vi "Periodic Tasks.vi"(8 "error in":errorcluster) -> ()   [LabVIEW 2018]
doc: "This VI runs in parallel to other tasks. It can contain as many user-defined periodic loops as you need. These can carry out PID or other sorts of timed response."
uses:
  <vilib>/Rock Robotics/WPI/ThirdParty/Phoenix-LabVIEW/Motor Controller/Controls/CTRE_Phoenix_MotorControl_ControlMode.ctl
  <vilib>/Rock Robotics/WPI/Utilities/WPI_GetSetVariantRefNum.vi
  <vilib>/Rock Robotics/Network Tables/NT Write Boolean Array.vi
  <vilib>/Rock Robotics/Network Tables/NT Write Numeric Array.vi
  <vilib>/Rock Robotics/WPI/Dashboard/Steer Command Global.vi
  <vilib>/Rock Robotics/WPI/Dashboard/Drive Command Global.vi
  Robot Global Data.vi
  <vilib>/Rock Robotics/Network Tables/NT Write Boolean.vi
  <vilib>/Rock Robotics/WPI/RobotDrive/WPI_RobotDriveMecanumDrive_Cartesian.vi
  <vilib>/Rock Robotics/WPI/ThirdParty/Phoenix-LabVIEW/Motor Controller/Get/CTRE_Phoenix_MotorController_GetAnalogData.vi
  <vilib>/Rock Robotics/Network Tables/NT Write Number.vi
  <vilib>/Rock Robotics/Network Tables/NT Read Number.vi
  <vilib>/Rock Robotics/WPI/Dashboard/Valid Target Global.vi
panel:
  out "TargetValid":bool
  out "DriveCommand":dbl(knob)=-0.0 scale=0.0..1.0
  in  "MaxDrive":dbl(slide)=0.20072992700729927 min=0.0 max=1.0 step=0.01 scale=0.0..1.0
  in  "DriveK":dbl(slide)=0.26277372262773724 min=0.0 max=1.0 step=0.05 scale=0.0..1.0
  in  "Limelight Goal Area":dbl(slide)=14.872262773722628 min=0.1 max=25.0 step=0.25 scale=0.0..25.0
  out "SteerCommand":dbl(knob) scale=-1.0..1.0
  in  "AimDeadband":dbl min=0.0 max=10.0 step=0.25
  in  "MinSteerCommand":dbl(slide)=0.02717391304347826 min=0.0 max=0.5 step=0.05 scale=0.0..0.5
  in  "SteeringK":dbl(slide)=0.007246376811594203 min=0.0 max=0.25 step=0.01 scale=0.0..0.25
  in  "Jack speed 3-2":dbl=-1.0
  in  "Jack drive 1-2":dbl=-0.75
  in  "Jack speed 2-2":dbl=1.0
  in  "Jack speed 1-2":dbl=1.0
  in  "Arm speed-2":dbl=-0.41
  in  "Pre Climb 2":i32=146
  in  "Load Cargo":i32=385
  in  "Arm speed":dbl=-0.55
  in  "Jack speed 1":dbl=1.0
  in  "Jack speed 2":dbl=1.0
  in  "Jack drive 1":dbl=-0.75
  in  "Jack speed 3":dbl=-1.0
  in  "Pre Climb":i32=80
  in  "Release Time":i32=7
  in  "Grab Drive Time":i32=7
  in  "Grab Wait Time":i32=2
  in  "Grab Time":i32=5
  in  "Home":i32=70
  in  "C High":i32=890
  in  "C Med":i32=540
  in  "C Low":i32=230
  in  "H High":i32=809
  in  "H Med":i32=475
  in  "H Low":i32=140
  out "Jack PO":dbl
  out "Arm PO":dbl
  out "Arm position":i32=55
  # "Climb 2 Case Values"
  # "Arm Actuators"
  # "Jack Mech."
  # "Jack Wheels"
  # "In pre climb cases add about 5% drive forward"
  # "Climb Case Values"
  # "Arm Actuators"
  # "Jack Mech."
  # "Jack Wheels"
  # "Grab and Release Times and Values\n                 In State Machine"
  # "State Machine Values for Positions"
  # "Proto Values Before Heartland"
  # "Pre Climb 2 146"
  # "H Low 171\nH Med 475\nH High 809"
  # "C Low 230\nC Med 540\nC High 890"
  # "Load Cargo 385\nHome 70\nPre Climb 80"
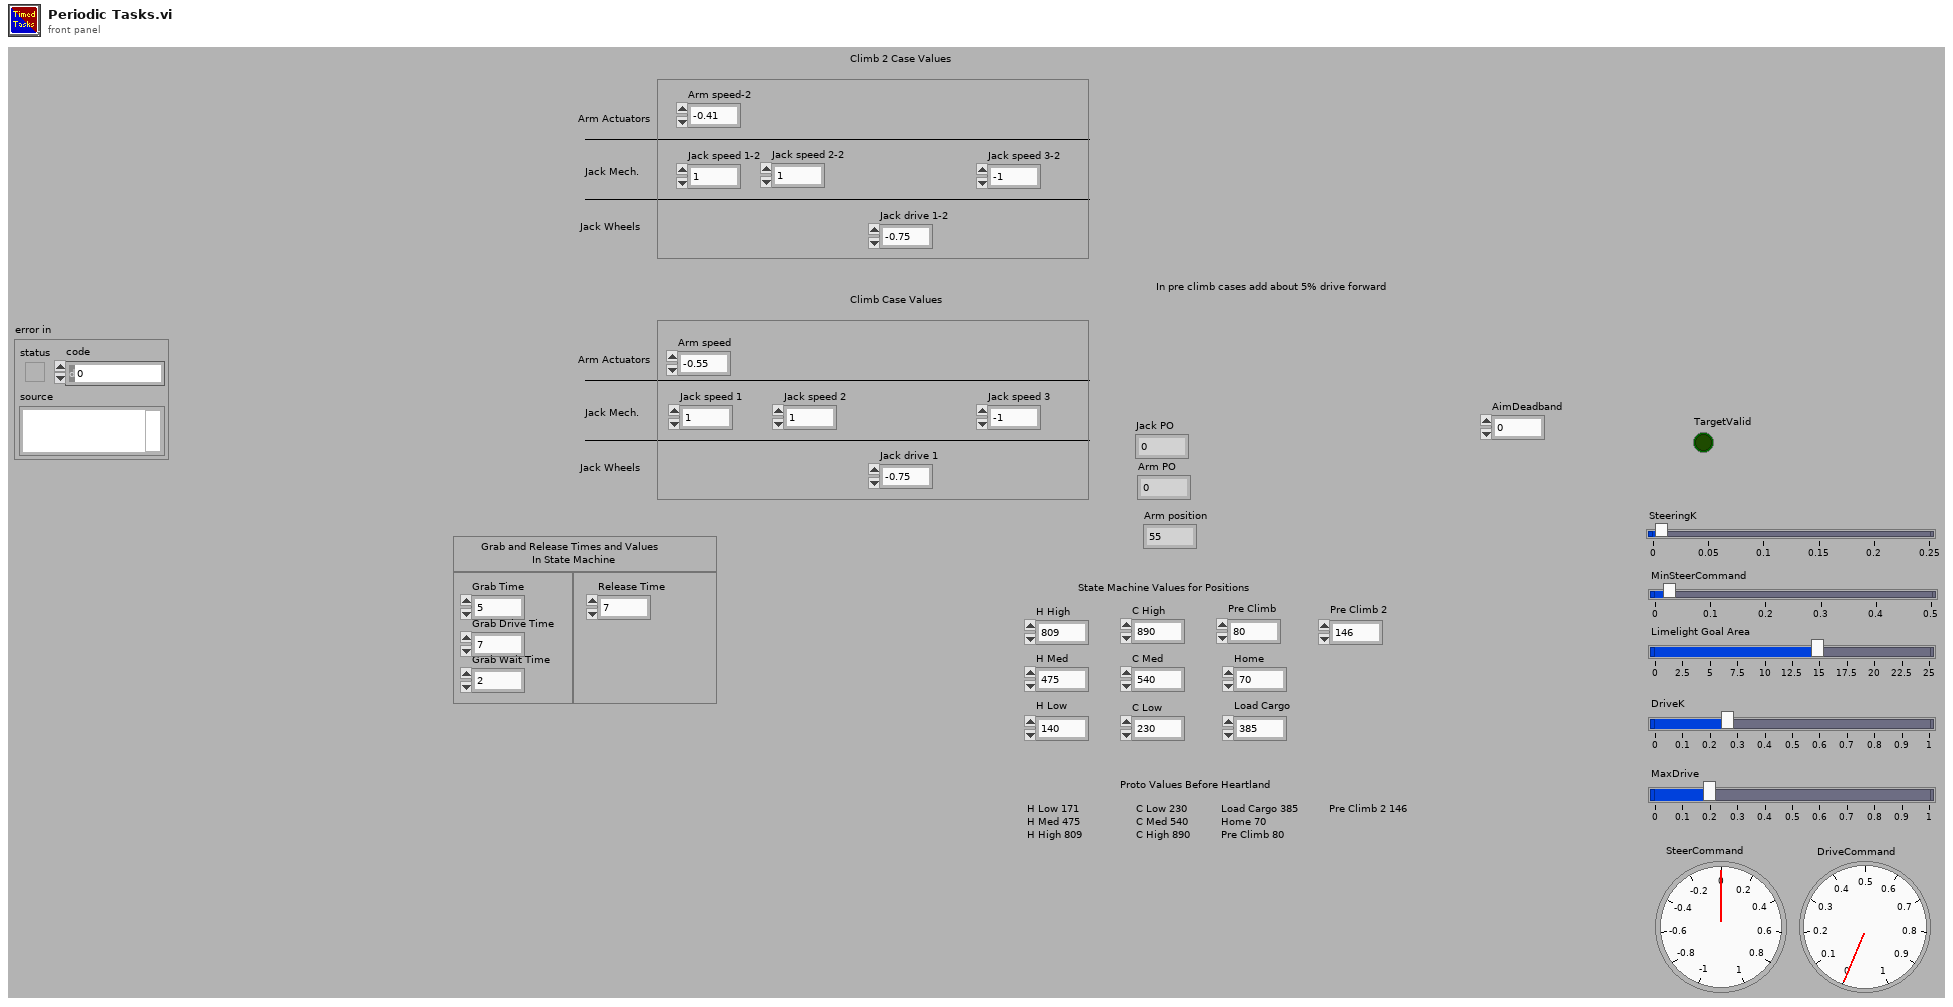
[diagram p1: front panel]
types:
  T1 = enum16{"Wait", "H.Low", "H.Med", "H.High", "C.Low", "C.Med", "C.High", "Home", "Pull Out Grab", "Pull Out Release", "Pre Climb", "Upward Travel", "Extra Jack Time", "Forward Travel", "Jack Retrieval", "Load Cargo", "Pre Climb 2", "Upward Travel 2", "Extra Jack Time 2", "Forward Travel 2", "Jack Retrieval 2"}
  T2 = typedef "WPI_DriverStationRobotMode2.ctl" = enum16{"Autonomous Disabled", "Autonomous Enabled", "Teleop Disabled", "Teleop Enabled", "Disconnected", "Finish", "Test Disabled", "Test Enabled", "Emergency Stopped"}
  T3 = typedef "WPI_MotorControlDeviceRef.ctl" = cluster{"DeviceStatus":errorcluster, "Type":T4, "PWM":cluster{"PWM Channel":T5, "DeadBand":T6}, "CAN":cluster{"Device Number":u8, "SetOutput VI Ref":variant, "GetOutput VI Ref":variant, "Enable VI Ref":variant, "Disable VI Ref":variant, "Data":variant}, "Invert":bool, "DIO PWM":cluster{"PWM \"Enable\" Channel":T5, "DIOChannel":T7, "PWM Rate":dbl}}
  T4 = typedef "WPI_MotorControlType.ctl" = enum16{"PWM", "CAN", "DIO PWM"}
  T5 = typedef "FPGA_DIOPWMChannel.ctl" = enum8{"PWM 0", "PWM 1", "PWM 2", "PWM 3", "PWM 4", "PWM 5", "PWM 6", "PWM 7", "PWM 8", "PWM 9", "PWM MXP 0", "PWM MXP 1", "PWM MXP 2", "PWM MXP 3", "PWM MXP 4", "PWM MXP 5", "PWM MXP 6", "PWM MXP 7", "PWM MXP 8", "PWM MXP 9", "Invalid"}
  T6 = typedef "WPI_PWMDeadband.ctl" = cluster{"Name":string, "maxPositivePwm":i32, "minPositivePwm":i32, "centerPwm":i32, "maxNegativePwm":i32, "minNegativePwm":i32, "angularRange":u16}
  T7 = typedef "FPGA_DIOChannel.ctl" = enum8{"DIO 0", "DIO 1", "DIO 2", "DIO 3", "DIO 4", "DIO 5", "DIO 6", "DIO 7", "DIO 8", "DIO 9", "DIO MXP 0", "DIO MXP 1", "DIO MXP 2", "DIO MXP 3", "DIO MXP 4", "DIO MXP 5", "DIO MXP 6", "DIO MXP 7", "DIO MXP 8", "DIO MXP 9", "DIO MXP 10", "DIO MXP 11", "DIO MXP 12", "DIO MXP 13", "DIO MXP 14", "DIO MXP 15", "SPI Port CS1", "SPI Port CS2", "SPI Port CS3", "SPI Port MISO", "SPI Port MOSI", "Invalid"}
  T8 = typedef "WPI_JoystickDevRef.ctl" = cluster{"Device":T9}
  T9 = typedef "WPI_JoystickDeviceEnum.ctl" = enum16{"USB 0", "USB 1", "USB 2", "USB 3", "USB 4", "USB 5"}
  T10 = typedef "CTRE_Phoenix_MotorControl_ControlMode.ctl" = u16
  T11 = typedef "WPI_RobotDriveDevRef.ctl" = cluster{"DevStatus":errorcluster, "Motors[]":T3[], "Square Inputs":bool, "Max Output":dbl}
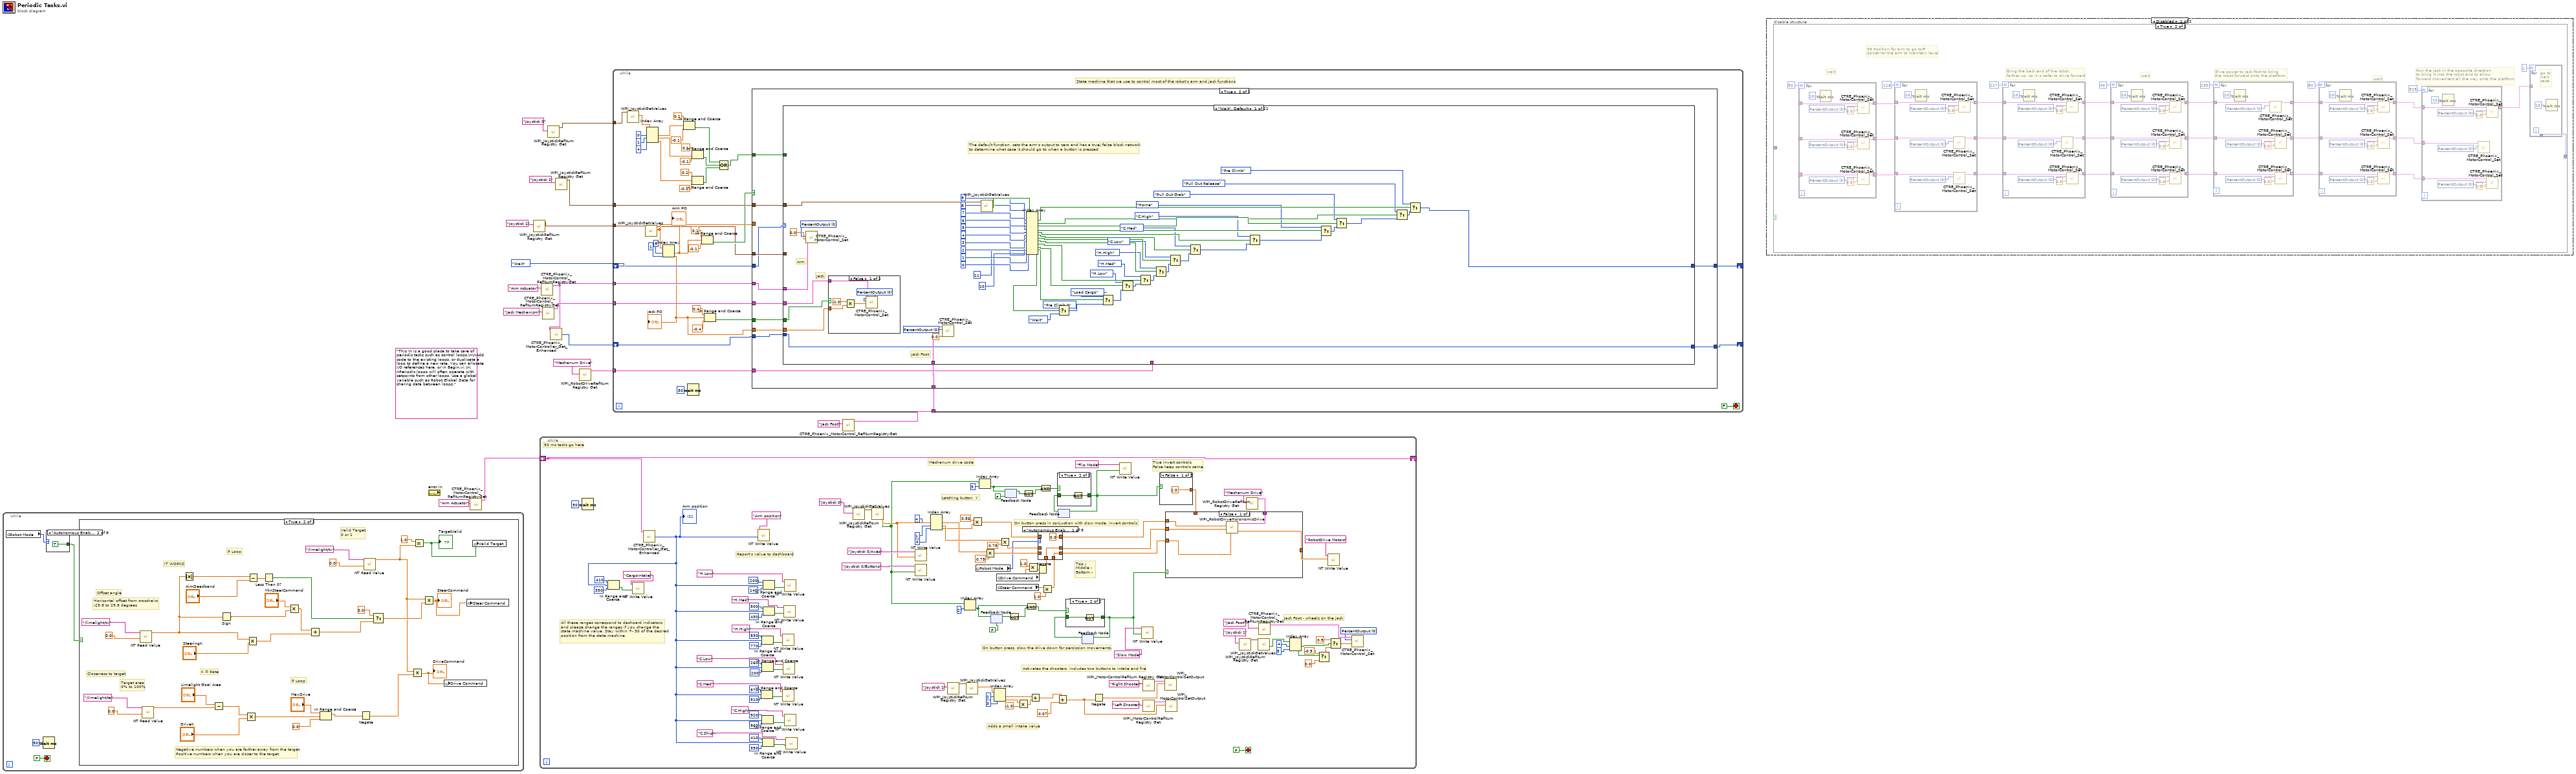
[diagram p0: block diagram]
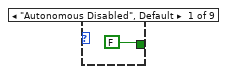
[diagram p2: hidden frame]
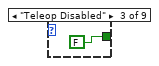
[diagram p3: hidden frame]
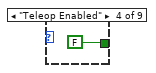
[diagram p4: hidden frame]
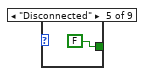
[diagram p5: hidden frame]
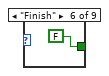
[diagram p6: hidden frame]
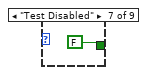
[diagram p7: hidden frame]
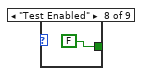
[diagram p8: hidden frame]
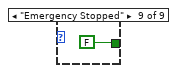
[diagram p9: hidden frame]
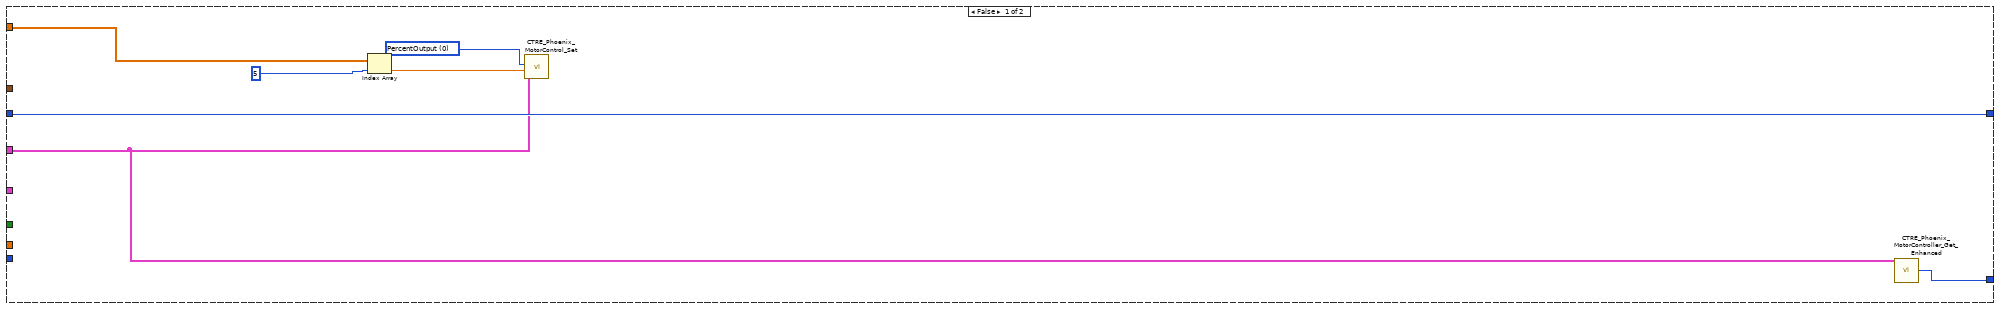
[diagram p13: hidden frame]
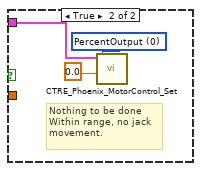
[diagram p14: hidden frame]
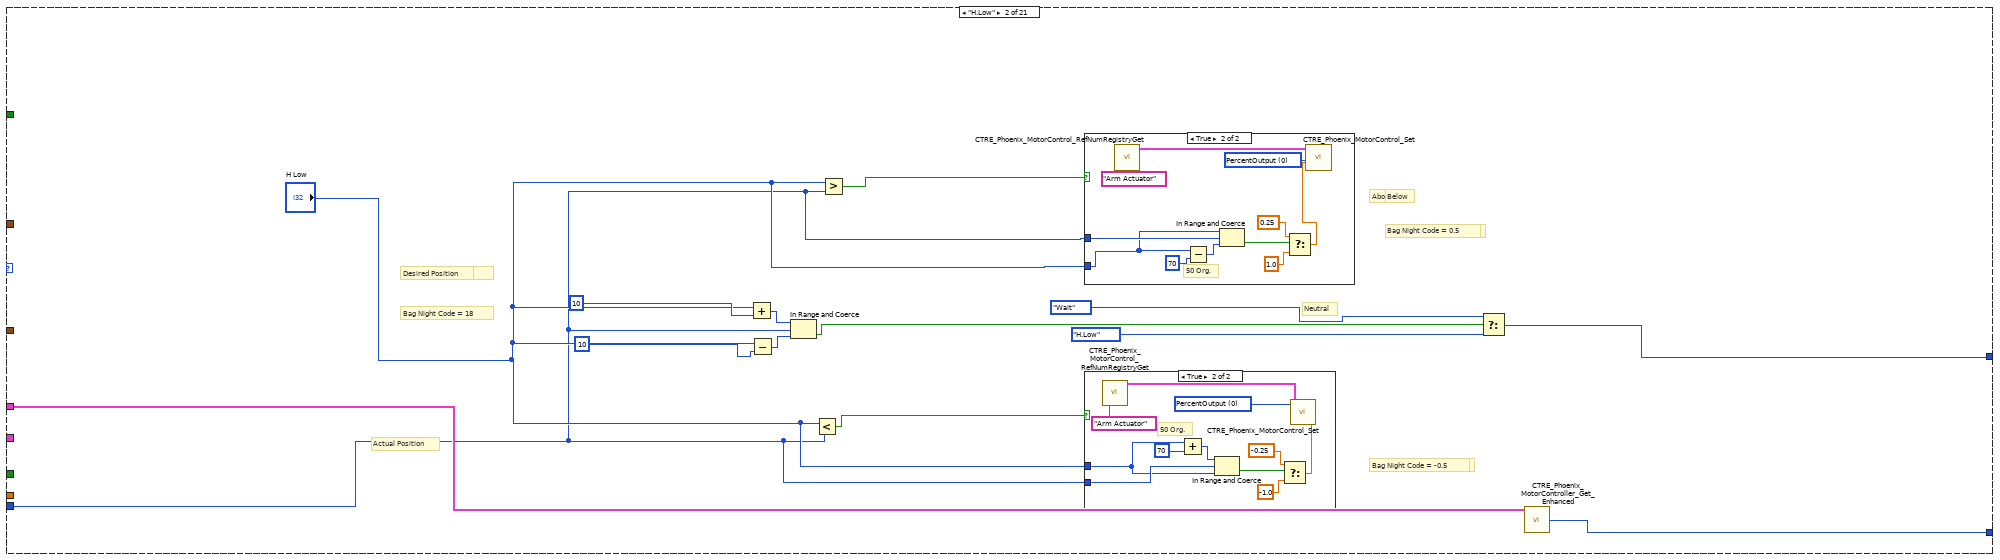
[diagram p15: hidden frame]
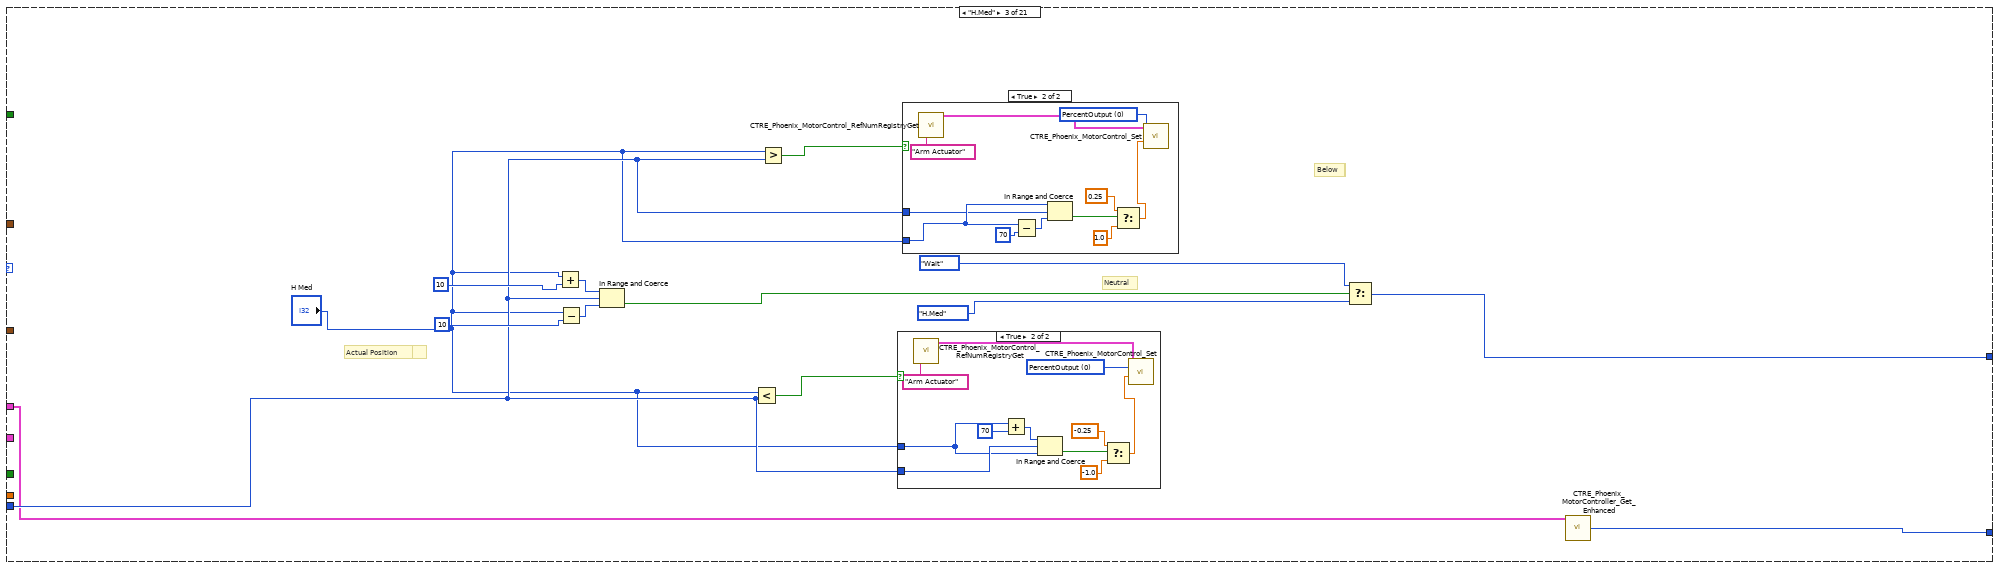
[diagram p18: hidden frame]
diagram:
  (unwired) "This VI is a good place to take care of periodic tasks such as control loops.\n\nAdd code to the existing loops, or duplicate a loop to define a new rate. You can allocate I/O references here, or in Begin.vi.\n\nPeriodic loops will often operate with setpoints from other loops. Use a global variable such as Robot Global Data for sharing data between loops."
  n1 = while {
    stop <- FALSE stop-if-true
    n2 = global read "Robot Global Data.vi" "Robot Mode"() -> (w21:T2)
    n3 = Wait (ms)(milliseconds to wait=u32 50) -> ()  [unwired: 1 out]
    n4 = case shown="\"Autonomous Enabled\"" w21 {
      tunnel: [FALSE TRUE FALSE FALSE FALSE FALSE FALSE FALSE FALSE] -> w22
      frame "Autonomous Disabled", Default {
      }
      frame "Autonomous Enabled" {
      }
      frame "Teleop Disabled" {
      }
      frame "Teleop Enabled" {
      }
      frame "Disconnected" {
      }
      frame "Finish" {
      }
      frame "Test Disabled" {
      }
      frame "Test Enabled" {
      }
      frame "Emergency Stopped" {
      }
    }
    n5 = case shown="True" w22 {
      frame False {
      }
      frame True {
        # "IT WORKS"
        # "Offset angle"
        # "Closeness to target"
        # "K = Rate"
        # "P Loop"
        # "P Loop"
        # "Negative numbers when you are farther away from the target\nPositive numbers when you are closer to the target"
        # "Valid Target\n0 or 1"
        # "Target area\n0% to 100%"
        # "Horizontal offset from crosshairs\n-29.8 to 29.8 degrees"
        n6 = call-poly <vilib>:"NT Read Value.vi"("Default Value"=0.0, "Name"="/limelight/tx") -> ("Numeric"=w38:dbl)  [unwired: 8 in, 1 out]
        n7 = call-poly <vilib>:"NT Read Value.vi"("Default Value"=0.0, "Name"="/limelight/ta") -> ("Numeric"=w46:dbl)  [unwired: 8 in, 1 out]
        n8 = Absolute Value(x=w38) -> (abs(x)=w60:dbl)
        n9 = Subtract(x="Limelight Goal Area", y=w46) -> (x-y=w44:dbl)
        n10 = Sign(1:w38) -> (0:w48:dbl)
        n11 = Multiply(x=w44, y="DriveK") -> (x*y=w43:dbl)
        n12 = Multiply(x=w38, y="SteeringK") -> (x*y=w57:dbl)
        n13 = Subtract(x=w60, y="AimDeadband") -> (x-y=w62:dbl)
        n14 = Less Than 0?(x=w62) -> (x < 0?=w63:bool)
        n15 = Multiply(x="MinSteerCommand", y=w48) -> (x*y=w59:dbl)
        n16 = Add(x=w59, y=w57) -> (x+y=w37:dbl)
        n17 = In Range and Coerce(upper limit="MaxDrive", x=w43, lower limit=0.0) -> (coerced(x)=w40:dbl)  [unwired: 1 out]
        n18 = Negate(x=w40) -> (-x=w39:dbl)
        n19 = call-poly <vilib>:"NT Read Value.vi"("Default Value"=0.0, "Name"="/limelight/tv") -> ("Numeric"=w36:dbl)  [unwired: 8 in, 1 out]
        n20 = Select(t=0.0, s=w63, f=w37) -> (s? t:f=w50:dbl)
        n21 = Multiply(x=w36, y=w39) -> (x*y=w32:dbl)
        "DriveCommand" <- w32
        n22 = Equal?(x=1.0, y=w36) -> (x = y?=w34:bool)
        "TargetValid" <- w34
        n23 = Multiply(x=w36, y=w50) -> (x*y=w33:dbl)
        "SteerCommand" <- w33
        n24 = global write "Drive Command Global.vi" "Drive Command"(w32) -> ()
        n25 = global write "Steer Command Global.vi" "Steer Command"(w33) -> ()
        n26 = global write "Valid Target Global.vi" "Valid Target"(w34) -> ()
      }
    }
  }
  n27 = call <vilib>:"CTRE_Phoenix_MotorControl_RefNumRegistryGet.vi"("refnum name"="Arm Actuator") -> ("PhoenixMotorControlDevRef"=w17:T3)  [unwired: 9 in, 1 out]
  n28 = call <vilib>:"WPI_JoystickRefNum Registry Get.vi"("refnum name"="Joystick 1") -> ("JoystickDevRef"=w13:T8)  [unwired: 9 in, 1 out]
  n29 = while {
    shift-right: [w113] -> _
    shift-left: w17 -> [w113]
    stop <- FALSE stop-if-true
    w90 = T10 0 items=["PercentOutput"=0, "Position"=1, "Velocity"=2, "Current"=3, "Follower"=5, "MotionProfile"=6, "MotionMagic"=7, "MotionProfileArc"=10, "Disabled"=15] ("Control Mode")
    # "Top -\nMiddle -\nBottom -"
    # "On button press in conjuction with slow mode, invert controls"
    # "Latching button  Y"
    # "True invert controls\nFalse keep controls same"
    # "Jack Foot - wheels on the jack"
    # "All these ranges correspond to dashoard indicators\nand please change the ranges if you change the \nstate machine value. Stay within +- 30 of the desired\nposition from the state machine."
    # "Adds a small intake value"
    # "On button press, slow the drive down for percission movements."
    # "Report's value to dashboard"
    # "Mechanum drive code"
    # "Activates the shooters, includes two buttons to intake and fire"
    # "50 ms tasks go here"
    n30 = Wait (ms)(milliseconds to wait=u32 50) -> ()  [unwired: 1 out]
    n31 = call-poly <vilib>:"CTRE_Phoenix_MotorController_Get_Enhanced.vi"("PhoenixMotorControlDevRef"=w113) -> ("AnalogInRaw"=w121:i32)  [unwired: 10 in, 4 out]
    "Arm position" <- w121
    n32 = In Range and Coerce(upper limit=410, x=w121, lower limit=350) -> (In Range?=w118:bool)  [unwired: 1 out]
    n33 = call-poly <vilib>:"NT Write Value.vi"("Boolean"=w118, "Name"="CargoIntake") -> ()  [unwired: 9 in, 1 out]
    n34 = call-poly <vilib>:"NT Write Value.vi"("Numeric"=w121, "Name"="Arm position") -> ()  [unwired: 9 in, 1 out]
    n35 = In Range and Coerce(upper limit=570, x=w121, lower limit=510) -> (In Range?=w136:bool)  [unwired: 1 out]
    n36 = In Range and Coerce(upper limit=260, x=w121, lower limit=200) -> (In Range?=w135:bool)  [unwired: 1 out]
    n37 = In Range and Coerce(upper limit=830, x=w121, lower limit=770) -> (In Range?=w134:bool)  [unwired: 1 out]
    n38 = In Range and Coerce(upper limit=920, x=w121, lower limit=860) -> (In Range?=w138:bool)  [unwired: 1 out]
    n39 = In Range and Coerce(upper limit=410, x=w121, lower limit=350) -> (In Range?=w137:bool)  [unwired: 1 out]
    n40 = In Range and Coerce(upper limit=200, x=w121, lower limit=140) -> (In Range?=w132:bool)  [unwired: 1 out]
    n41 = In Range and Coerce(upper limit=500, x=w121, lower limit=430) -> (In Range?=w133:bool)  [unwired: 1 out]
    n42 = call-poly <vilib>:"NT Write Value.vi"("Boolean"=w134, "Name"="H.High") -> ()  [unwired: 9 in, 1 out]
    n43 = call-poly <vilib>:"NT Write Value.vi"("Boolean"=w136, "Name"="C.Med") -> ()  [unwired: 9 in, 1 out]
    n44 = call-poly <vilib>:"NT Write Value.vi"("Boolean"=w135, "Name"="C.Low") -> ()  [unwired: 9 in, 1 out]
    n45 = call-poly <vilib>:"NT Write Value.vi"("Boolean"=w133, "Name"="H.Med") -> ()  [unwired: 9 in, 1 out]
    n46 = call-poly <vilib>:"NT Write Value.vi"("Boolean"=w132, "Name"="H.Low") -> ()  [unwired: 9 in, 1 out]
    n47 = call-poly <vilib>:"NT Write Value.vi"("Boolean"=w138, "Name"="C.High") -> ()  [unwired: 9 in, 1 out]
    n48 = call-poly <vilib>:"NT Write Value.vi"("Boolean"=w137, "Name"="C.Ship") -> ()  [unwired: 9 in, 1 out]
    n49 = call <vilib>:"WPI_JoystickRefNum Registry Get.vi"("refnum name"="Joystick 0") -> ("JoystickDevRef"=w183:T8)  [unwired: 1 in, 9 out]
    n50 = call <vilib>:"WPI_JoystickGetValues.vi"("JoystickDevRef"=w183) -> ("Buttons"=w80:bool[], "Axes"=w180:dbl[])  [unwired: 6 in, 3 out]
    n51 = call-poly <vilib>:"NT Write Value.vi"("Numeric Array"=w180, "Name"="Joystick 0/Axes") -> ()  [unwired: 9 in, 1 out]
    n52 = call-poly <vilib>:"NT Write Value.vi"("Boolean Array"=w80, "Name"="Joystick 0/Buttons") -> ()  [unwired: 9 in, 1 out]
    n53 = Index Array(array=w180, index #1=4 ("index"), index #2=1 ("index"), index #3=0 ("index")) -> (element #1=w114:dbl, element #2=w162:dbl, element #3=w115:dbl)
    n54 = call <vilib>:"WPI_JoystickRefNum Registry Get.vi"("refnum name"="Joystick 1") -> ("JoystickDevRef"=w179:T8)  [unwired: 1 in, 9 out]
    n55 = Index Array(array=w80, index=2) -> (element=w109:bool)
    n56 = call <vilib>:"WPI_JoystickGetValues.vi"("JoystickDevRef"=w179) -> ("Axes"=w173:dbl[])  [unwired: 6 in, 4 out]
    n57 = Multiply(x=0.56, y=w115) -> (x*y=w73:dbl)
    n58 = global read "Robot Global Data.vi" "Robot Mode"() -> (w71:T2)
    n59 = Index Array(array=w80, index=3) -> (element=w84:bool)
    n60 = Multiply(x=w114, y=0.75) -> (x*y=w78:dbl)
    n61 = feedback-in #1(w109) -> ()
    n62 = feedback #1(FALSE) -> (w111:bool)
    n63 = Index Array(array=w173, index #1=2 ("index"), index #2=3 ("index")) -> (element #1=w167:dbl, element #2=w169:dbl)
    n64 = global read "Drive Command Global.vi" "Drive Command"() -> (w72:dbl)
    n65 = global read "Steer Command Global.vi" "Steer Command"() -> (w69:dbl)
    n66 = Multiply(x=w162, y=0.75) -> (x*y=w76:dbl)
    n67 = feedback #2(FALSE) -> (w86:bool)
    n68 = feedback-in #2(w84) -> ()
    n69 = Not(x=w111) -> (.not. x?=w110:bool)
    n70 = Multiply(x=w169, y=-1.0) -> (x*y=w168:dbl)
    n71 = Not(x=w86) -> (.not. x?=w85:bool)
    n72 = And(x=w109, y=w110) -> (x .and. y?=w108:bool)
    n73 = Multiply(x=1.0, y=w72) -> (x*y=w66:dbl)
    n74 = Add(x=w167, y=w168) -> (x+y=w156:dbl)
    n75 = Negate(x=w66) -> (-x=w70:dbl)
    n76 = And(x=w84, y=w85) -> (x .and. y?=w83:bool)
    n77 = Multiply(x=w69, y=1.0) -> (x*y=w68:dbl)
    n78 = case shown="\"Autonomous Enabled\"" w71 {
      tunnel: w78 -> [_ w189 w192 w195 w198 w201 w204 w207 w210]
      tunnel: [w187 w189 w192 w195 w198 w201 w204 w207 w210] -> w77
      tunnel: w76 -> [_ w190 w193 w196 w199 w202 w205 w208 w211]
      tunnel: [w188 w190 w193 w196 w199 w202 w205 w208 w211] -> w75
      tunnel: w73 -> [_ w191 w194 w197 w200 w203 w206 w209 w212]
      tunnel: [0.0 w191 w194 w197 w200 w203 w206 w209 w212] -> w74
      tunnel: w70 -> [w188 _ _ _ _ _ _ _ _]
      tunnel: w68 -> [w187 _ _ _ _ _ _ _ _]
      frame "Autonomous Enabled" {
      }
      frame "Teleop Enabled" {
      }
      frame "Disconnected" {
      }
      frame "Finish" {
      }
      frame "Test Disabled" {
      }
      frame "Test Enabled" {
      }
      frame "Emergency Stopped" {
      }
      frame "Teleop Disabled" {
      }
      frame "Autonomous Disabled" {
      }
    }
    n79 = Add(x=w156, y=0.07) -> (x+y=w154:dbl)
    n80 = feedback #3() -> (w82:bool)  [unwired: 1 in]
    n81 = case shown="True" w83 {
      tunnel: w82 -> [w213 w215]
      tunnel: [w213 w214] -> w79
      frame False {
      }
      frame True {
        n82 = Not(x=w215) -> (.not. x?=w214:bool)
      }
    }
    n83 = feedback-in #3(w79) -> ()
    n84 = feedback #4() -> (w107:bool)  [unwired: 1 in]
    n85 = case shown="True" w108 {
      tunnel: w107 -> [w218 w220]
      tunnel: [w218 w219] -> w106
      frame False {
      }
      frame True {
        n86 = Not(x=w220) -> (.not. x?=w219:bool)
      }
    }
    n87 = feedback-in #4(w106) -> ()
    n88 = Negate(x=w154) -> (-x=w166:dbl)
    n89 = call-poly <vilib>:"NT Write Value.vi"("Boolean"=w79, "Name"="Flip Mode") -> ()  [unwired: 9 in, 1 out]
    n90 = call-poly <vilib>:"NT Write Value.vi"("Boolean"=w106, "Name"="Slow Mode") -> ()  [unwired: 9 in, 1 out]
    n91 = call <vilib>:"WPI_MotorControlRefNum Registry Get.vi"("refnum name"="Right Shooter") -> ("MotorControlDevRef"=w175:T3)  [unwired: 9 in, 1 out]
    n92 = call <vilib>:"WPI_MotorControlRefNum Registry Get.vi"("refnum name"="Left Shooter") -> ("MotorControlDevRef"=w174:T3)  [unwired: 9 in, 1 out]
    n93 = case shown="False" w79 {
      tunnel: [1.0 -1.0] -> w89
      frame False {
      }
      frame True {
      }
    }
    n94 = call <vilib>:"WPI_MotorControlSetOutput.vi"("Output"=w166, "MotorControlDevRef"=w175) -> ()  [unwired: 7 in, 3 out]
    n95 = call <vilib>:"WPI_MotorControlSetOutput.vi"("Output"=w154, "MotorControlDevRef"=w174) -> ()  [unwired: 7 in, 3 out]
    n96 = call <vilib>:"WPI_JoystickRefNum Registry Get.vi"("refnum name"="Joystick 1") -> ("JoystickDevRef"=w103:T8)  [unwired: 1 in, 9 out]
    n97 = call <vilib>:"WPI_RobotDriveRefNum Registry Get.vi"("refnum name"="Mechanum Drive") -> ("RobotDriveDevRef"=w163:T11)  [unwired: 1 in, 9 out]
    n98 = case shown="False" w106 {
      tunnel: w163 -> [w223 w239]
      tunnel: [w224 w238] -> w161
      tunnel: w74 -> [w221 w230]
      tunnel: w75 -> [w225 w233]
      tunnel: w77 -> [w222 w226]
      tunnel: w89 -> [_ w227]
      frame False {
        n99 = call-poly <vilib>:"WPI_RobotDriveHolonomicDrive.vi"("Rotation"=w222, "Y"=w225, "X"=w221, "RobotDriveDevRef"=w223) -> ("Motor Values"=w224:dbl[])  [unwired: 5 in, 2 out]
      }
      frame True {
        n100 = Multiply(x=w233, y=w227) -> (x*y=w229:dbl)
        n101 = Multiply(x=w230, y=w227) -> (x*y=w228:dbl)
        n102 = Multiply(x=w226, y=0.25 ("x")) -> (x*y=w237:dbl)
        n103 = Multiply(x=w229, y=0.25) -> (x*y=w235:dbl)
        n104 = Multiply(x=w228, y=0.25 ("x")) -> (x*y=w232:dbl)
        n105 = call-poly <vilib>:"WPI_RobotDriveHolonomicDrive.vi"("Rotation"=w237, "Y"=w235, "X"=w232, "RobotDriveDevRef"=w239) -> ("Motor Values"=w238:dbl[])  [unwired: 5 in, 2 out]
      }
    }
    n106 = call <vilib>:"WPI_JoystickGetValues.vi"("JoystickDevRef"=w103) -> ("Buttons"=w100:bool[])  [unwired: 6 in, 4 out]
    n107 = call <vilib>:"CTRE_Phoenix_MotorControl_RefNumRegistryGet.vi"("refnum name"="Jack Foot") -> ("PhoenixMotorControlDevRef"=w93:T3)  [unwired: 9 in, 1 out]
    n108 = Index Array(array=w100, index #1=4 ("index"), index #2=5 ("index")) -> (element #1=w98:bool, element #2=w99:bool)
    n109 = Select(t=-0.5, s=w99, f=0.0) -> (s? t:f=w97:dbl)
    n110 = call-poly <vilib>:"NT Write Value.vi"("Numeric Array"=w161, "Name"="RobotDrive Motors") -> ()  [unwired: 9 in, 1 out]
    n111 = Select(t=0.5, s=w98, f=w97) -> (s? t:f=w91:dbl)
    n112 = call <vilib>:"CTRE_Phoenix_MotorControl_Set.vi"("Output"=w91, "Control Mode"=w90, "PhoenixMotorControlDevRef"=w93) -> ()  [unwired: 7 in, 2 out]
  }
  n113 = call <vilib>:"CTRE_Phoenix_MotorControl_RefNumRegistryGet.vi"("refnum name"="Arm Actuator") -> ("PhoenixMotorControlDevRef"=w6:T3)  [unwired: 9 in, 1 out]
  n114 = call <vilib>:"CTRE_Phoenix_MotorControl_RefNumRegistryGet.vi"("refnum name"="Jack Mechanism") -> ("PhoenixMotorControlDevRef"=w9:T3)  [unwired: 9 in, 1 out]
  n115 = call <vilib>:"WPI_JoystickRefNum Registry Get.vi"("refnum name"="Joystick 0") -> ("JoystickDevRef"=w11:T8)  [unwired: 9 in, 1 out]
  n116 = call-poly <vilib>:"CTRE_Phoenix_MotorController_Get_Enhanced.vi"("PhoenixMotorControlDevRef"=w6) -> ("AnalogInRaw"=w3:i32)  [unwired: 10 in, 4 out]
  n117 = call <vilib>:"WPI_JoystickRefNum Registry Get.vi"("refnum name"="Joystick 2") -> ("JoystickDevRef"=w4:T8)  [unwired: 9 in, 1 out]
  n118 = call <vilib>:"WPI_RobotDriveRefNum Registry Get.vi"("refnum name"="Mechanum Drive") -> ("RobotDriveDevRef"=w7:T11)  [unwired: 1 in, 9 out]
  n119 = call <vilib>:"CTRE_Phoenix_MotorControl_RefNumRegistryGet.vi"("refnum name"="Jack Foot") -> ("PhoenixMotorControlDevRef"=w1:T3)  [unwired: 9 in, 1 out]
  n120 = while {
    shift-right: [w257] -> _
    shift-left: T1."Wait" -> [w241]
    tunnel: w13 -> [w280]
    tunnel: w6 -> [w275]
    tunnel: w11 -> [w258]
    tunnel: w9 -> [w252]
    tunnel: w7 -> [w251]
    tunnel: w4 -> [w250]
    shift-right: [w248] -> _
    shift-left: w3 -> [w249]
    tunnel: w1 -> [w243]
    stop <- FALSE stop-if-true
    # "State machine that we use to control most of the robot's arm and jack functions"
    n121 = call <vilib>:"WPI_JoystickGetValues.vi"("JoystickDevRef"=w258) -> ("Axes"=w267:dbl[])  [unwired: 6 in, 4 out]
    n122 = call <vilib>:"WPI_JoystickGetValues.vi"("JoystickDevRef"=w280) -> ("Axes"=w274:dbl[], "JoystickDevRef"=w273:T8)  [unwired: 6 in, 3 out]
    n123 = Index Array(array=w267, index #1=0 ("index"), index #2=1 ("index"), index #3=4 ("index")) -> (element #1=w268:dbl, element #2=w260:dbl, element #3=w259:dbl)
    n124 = Index Array(array=w274, index #1=5 ("index"), index #2=1 ("index")) -> (element #1=w277:dbl, element #2=w240:dbl)
    "Jack PO" <- w240
    "Arm PO" <- w277
    n125 = In Range and Coerce(upper limit=0.1, x=w268, lower limit=-0.1) -> (In Range?=w245:bool)  [unwired: 1 out]
    n126 = Wait (ms)(milliseconds to wait=u32 50) -> ()  [unwired: 1 out]
    n127 = In Range and Coerce(upper limit=0.1, x=w260, lower limit=-0.1) -> (In Range?=w247:bool)  [unwired: 1 out]
    n128 = In Range and Coerce(upper limit=0.1, x=w259, lower limit=-0.1) -> (In Range?=w246:bool)  [unwired: 1 out]
    n129 = In Range and Coerce(upper limit=0.1, x=w277, lower limit=-0.1) -> (In Range?=w276:bool)  [unwired: 1 out]
    n130 = In Range and Coerce(upper limit=0.4, x=w240, lower limit=-0.4) -> (In Range?=w253:bool)  [unwired: 1 out]
    n131 = Compound Arithmetic op=OR(w245, w247, w246) -> (w244:bool)
    n132 = case shown="True" w276 {
      tunnel: w241 -> [w284 w290]
      tunnel: w275 -> [w282 w301]
      tunnel: w274 -> [w285 _]
      tunnel: w273 -> [_ w300]
      tunnel: w244 -> [_ w299]
      tunnel: [w284 w298] -> w257
      tunnel: w253 -> [_ w297]
      tunnel: w252 -> [_ w296]
      tunnel: w251 -> [_ w295]
      tunnel: w249 -> [_ w293]
      tunnel: w250 -> [_ w294]
      tunnel: [w283 w292] -> w248
      tunnel: w243 -> [_ w291]
      tunnel: w240 -> [_ w289]
      frame False {
        w288 = T10 0 items=["PercentOutput"=0, "Position"=1, "Velocity"=2, "Current"=3, "Follower"=5, "MotionProfile"=6, "MotionMagic"=7, "MotionProfileArc"=10, "Disabled"=15] ("Control Mode")
        n133 = Index Array(array=w285, index=5) -> (element=w286:dbl)
        n134 = call <vilib>:"CTRE_Phoenix_MotorControl_Set.vi"("Output"=w286, "Control Mode"=w288, "PhoenixMotorControlDevRef"=w282) -> ()  [unwired: 7 in, 2 out]
        n135 = call-poly <vilib>:"CTRE_Phoenix_MotorController_Get_Enhanced.vi"("PhoenixMotorControlDevRef"=w282) -> ("AnalogInRaw"=w283:i32)  [unwired: 10 in, 4 out]
      }
      frame True {
        n136 = case shown="\"Wait\", Default" w290 {
          selector: w290 -> [_ _ _ _ _ _ _ _ w627 w654 _ _ _ _ _ _ _ _ _ _ _]
          tunnel: w301 -> [w362 w375 w409 w447 w483 w519 w555 w591 w623 w649 w676 w715 w737 w759 w781 w801 w834 w875 w897 w920 w946]
          tunnel: w300 -> [_ _ _ _ _ _ _ _ _ _ _ _ _ _ _ _ _ _ _ _ _]
          tunnel: w299 -> [_ _ _ _ _ _ _ _ w628 w653 _ _ _ _ _ _ _ _ _ _ _]
          tunnel: [w326 w377 w413 w450 w485 w521 w559 w593 w626 w652 w674 w709 w731 w754 w776 w799 w833 w868 w891 w914 w940] -> w298
          tunnel: w297 -> [w302 _ _ _ _ _ _ _ _ _ _ _ _ _ _ _ _ _ _ _ _]
          tunnel: w296 -> [w304 _ _ _ _ _ _ _ _ _ _ w712 w736 w758 w780 _ _ w874 w896 w919 w945]
          tunnel: w295 -> [_ _ _ _ _ _ _ _ w625 w651 _ _ _ _ _ _ _ _ _ w913 _]
          tunnel: w293 -> [w328 w373 w411 w446 w482 w518 w554 w590 _ _ w675 w716 w738 w760 w782 w800 w835 w877 w899 w922 w948]
          tunnel: w294 -> [w350 _ _ _ _ _ _ _ _ _ _ _ _ _ _ _ _ _ _ _ _]
          tunnel: [w328 w376 w412 w448 w484 w520 w556 w592 w624 w650 w673 w716 w738 w760 w782 w798 w832 w877 w899 w922 w948] -> w292
          tunnel: w291 -> [w307 _ _ _ _ _ _ _ _ _ _ w711 w735 w757 w779 _ _ w873 w895 w918 w944]
          tunnel: w289 -> [w303 _ _ _ _ _ _ _ _ _ _ _ _ _ _ _ _ _ _ _ _]
          frame "Wait", Default {
            w306 = T10 0 items=["PercentOutput"=0, "Position"=1, "Velocity"=2, "Current"=3, "Follower"=5, "MotionProfile"=6, "MotionMagic"=7, "MotionProfileArc"=10, "Disabled"=15] ("Control Mode")
            w361 = T10 0 items=["PercentOutput"=0, "Position"=1, "Velocity"=2, "Current"=3, "Follower"=5, "MotionProfile"=6, "MotionMagic"=7, "MotionProfileArc"=10, "Disabled"=15] ("Control Mode")
            # "Jack Foot"
            # "Jack"
            # "Arm"
            # "The default function, sets the arm's output to zero and has a true/ false block network\nto determine what case it should go to when a button is pressed"
            n137 = call <vilib>:"CTRE_Phoenix_MotorControl_Set.vi"("Output"=0.0, "Control Mode"=w361, "PhoenixMotorControlDevRef"=w362) -> ()  [unwired: 7 in, 2 out]
            n138 = case shown="False" w302 {
              tunnel: w304 -> [w363 w370]
              tunnel: w303 -> [w364 _]
              frame False {
                w365 = T10 0 items=["PercentOutput"=0, "Position"=1, "Velocity"=2, "Current"=3, "Follower"=5, "MotionProfile"=6, "MotionMagic"=7, "MotionProfileArc"=10, "Disabled"=15] ("Control Mode")
                n139 = Multiply(x=-1.0, y=w364) -> (x*y=w367:dbl)
                n140 = call <vilib>:"CTRE_Phoenix_MotorControl_Set.vi"("Output"=w367, "Control Mode"=w365, "PhoenixMotorControlDevRef"=w363) -> ()  [unwired: 7 in, 2 out]
              }
              frame True {
                w369 = T10 0 items=["PercentOutput"=0, "Position"=1, "Velocity"=2, "Current"=3, "Follower"=5, "MotionProfile"=6, "MotionMagic"=7, "MotionProfileArc"=10, "Disabled"=15] ("Control Mode")
                # "Nothing to be done\nWithin range, no jack\nmovement."
                n141 = call <vilib>:"CTRE_Phoenix_MotorControl_Set.vi"("Output"=0.0 ("x"), "Control Mode"=w369, "PhoenixMotorControlDevRef"=w370) -> ()  [unwired: 7 in, 2 out]
              }
            }
            n142 = call <vilib>:"CTRE_Phoenix_MotorControl_Set.vi"("Output"=0.0, "Control Mode"=w306, "PhoenixMotorControlDevRef"=w307) -> ()  [unwired: 7 in, 2 out]
            n143 = call <vilib>:"WPI_JoystickGetValues.vi"("JoystickDevRef"=w350) -> ("Buttons"=w349:bool[])  [unwired: 6 in, 4 out]
            n144 = Index Array(array=w349, index #1=9 ("index"), index #2=8 ("index"), index #3=7 ("index"), index #4=6 ("index"), index #5=5 ("index"), index #6=4 ("index"), index #7=3 ("index"), index #8=2 ("index"), index #9=1 ("index"), index #10=0 ("index"), index #11=11 ("index"), index #12=10 ("index")) -> (element #1=w339:bool, element #2=w340:bool, element #3=w341:bool, element #4=w342:bool, element #5=w343:bool, element #6=w344:bool, element #7=w345:bool, element #8=w346:bool, element #9=w347:bool, element #10=w348:bool, element #11=w324:bool, element #12=w322:bool)
            n145 = Select(t=T1."Pre Climb 2", s=w322, f=T1."Wait") -> (s? t:f=w323:T1)
            n146 = Select(t=T1."Load Cargo", s=w324, f=w323) -> (s? t:f=w325:T1)
            n147 = Select(t=T1."H.Low", s=w348, f=w325) -> (s? t:f=w359:T1)
            n148 = Select(t=T1."H.Med", s=w347, f=w359) -> (s? t:f=w358:T1)
            n149 = Select(t=T1."H.High", s=w346, f=w358) -> (s? t:f=w357:T1)
            n150 = Select(t=T1."C.Low", s=w345, f=w357) -> (s? t:f=w356:T1)
            n151 = Select(t=T1."C.Med", s=w344, f=w356) -> (s? t:f=w355:T1)
            n152 = Select(t=T1."C.High", s=w343, f=w355) -> (s? t:f=w354:T1)
            n153 = Select(t=T1."Home", s=w342, f=w354) -> (s? t:f=w353:T1)
            n154 = Select(t=T1."Pull Out Grab", s=w341, f=w353) -> (s? t:f=w352:T1)
            n155 = Select(t=T1."Pull Out Release", s=w340, f=w352) -> (s? t:f=w351:T1)
            n156 = Select(t=T1."Pre Climb", s=w339, f=w351) -> (s? t:f=w326:T1)
          }
          frame "H.Low" {
            # "Bag Night Code = 0.5"
            # "Bag Night Code = 0.75"
            # "Bag Night Code = -0.5"
            # "Bag Night Code = -0.75"
            # "Bag Night Code = 18"
            # "Bag Night Code = 18"
            # "Actual Position"
            # "Desired Position"
            # "Below"
            # "Neutral"
            # "Above"
            n157 = Add(x="H Low", y=10) -> (x+y=w382:i32)
            n158 = Subtract(x="H Low", y=10) -> (x-y=w383:i32)
            n159 = In Range and Coerce(upper limit=w382, x=w373, lower limit=w383) -> (In Range?=w378:bool)  [unwired: 1 out]
            n160 = Less?(x="H Low", y=w373) -> (x < y?=w380:bool)
            n161 = Greater?(x="H Low", y=w373) -> (0:w379:bool)
            n162 = case shown="True" w379 {
              tunnel: "H Low" -> [_ w396]
              tunnel: w373 -> [_ w397]
              frame False {
              }
              frame True {
                w404 = T10 0 items=["PercentOutput"=0, "Position"=1, "Velocity"=2, "Current"=3, "Follower"=5, "MotionProfile"=6, "MotionMagic"=7, "MotionProfileArc"=10, "Disabled"=15] ("Control Mode")
                # "50 Org."
                n163 = call <vilib>:"CTRE_Phoenix_MotorControl_RefNumRegistryGet.vi"("refnum name"="Arm Actuator") -> ("PhoenixMotorControlDevRef"=w406:T3)  [unwired: 9 in, 1 out]
                n164 = Subtract(x=w396, y=70) -> (x-y=w400:i32)
                n165 = In Range and Coerce(upper limit=w396, x=w397, lower limit=w400) -> (In Range?=w399:bool)  [unwired: 1 out]
                n166 = Select(t=0.25 ("Output"), s=w399, f=1.0 ("Output")) -> (s? t:f=w398:dbl)
                n167 = call <vilib>:"CTRE_Phoenix_MotorControl_Set.vi"("Output"=w398, "Control Mode"=w404, "PhoenixMotorControlDevRef"=w406) -> ()  [unwired: 7 in, 2 out]
              }
            }
            n168 = case shown="True" w380 {
              tunnel: "H Low" -> [_ w385]
              tunnel: w373 -> [_ w386]
              frame False {
              }
              frame True {
                w393 = T10 0 items=["PercentOutput"=0, "Position"=1, "Velocity"=2, "Current"=3, "Follower"=5, "MotionProfile"=6, "MotionMagic"=7, "MotionProfileArc"=10, "Disabled"=15] ("Control Mode")
                # "50 Org."
                n169 = call <vilib>:"CTRE_Phoenix_MotorControl_RefNumRegistryGet.vi"("refnum name"="Arm Actuator") -> ("PhoenixMotorControlDevRef"=w395:T3)  [unwired: 9 in, 1 out]
                n170 = Add(x=w385, y=70) -> (x+y=w389:i32)
                n171 = In Range and Coerce(upper limit=w389, x=w386, lower limit=w385) -> (In Range?=w387:bool)  [unwired: 1 out]
                n172 = Select(t=-0.25 ("Output"), s=w387, f=-1.0 ("Output")) -> (s? t:f=w392:dbl)
                n173 = call <vilib>:"CTRE_Phoenix_MotorControl_Set.vi"("Output"=w392, "Control Mode"=w393, "PhoenixMotorControlDevRef"=w395) -> ()  [unwired: 7 in, 2 out]
              }
            }
            n174 = Select(t=T1."Wait", s=w378, f=T1."H.Low") -> (s? t:f=w377:T1)
            n175 = call-poly <vilib>:"CTRE_Phoenix_MotorController_Get_Enhanced.vi"("PhoenixMotorControlDevRef"=w375) -> ("AnalogInRaw"=w376:i32)  [unwired: 10 in, 4 out]
          }
          frame "H.Med" {
            # "Actual Position"
            # "Desired Position"
            # "Below"
            # "Neutral"
            # "Above"
            n176 = Add(x="H Med", y=10) -> (x+y=w418:i32)
            n177 = Subtract(x="H Med", y=10) -> (x-y=w419:i32)
            n178 = In Range and Coerce(upper limit=w418, x=w411, lower limit=w419) -> (In Range?=w414:bool)  [unwired: 1 out]
            n179 = Less?(x="H Med", y=w411) -> (x < y?=w416:bool)
            n180 = Greater?(x="H Med", y=w411) -> (0:w415:bool)
            n181 = case shown="True" w416 {
              tunnel: w411 -> [_ w423]
              tunnel: "H Med" -> [_ w422]
              frame False {
              }
              frame True {
                w429 = T10 0 items=["PercentOutput"=0, "Position"=1, "Velocity"=2, "Current"=3, "Follower"=5, "MotionProfile"=6, "MotionMagic"=7, "MotionProfileArc"=10, "Disabled"=15] ("Control Mode")
                n182 = call <vilib>:"CTRE_Phoenix_MotorControl_RefNumRegistryGet.vi"("refnum name"="Arm Actuator") -> ("PhoenixMotorControlDevRef"=w431:T3)  [unwired: 9 in, 1 out]
                n183 = Add(x=w422, y=70) -> (x+y=w426:i32)
                n184 = In Range and Coerce(upper limit=w426, x=w423, lower limit=w422) -> (In Range?=w424:bool)  [unwired: 1 out]
                n185 = Select(t=-0.25 ("Output"), s=w424, f=-1.0 ("Output")) -> (s? t:f=w421:dbl)
                n186 = call <vilib>:"CTRE_Phoenix_MotorControl_Set.vi"("Output"=w421, "Control Mode"=w429, "PhoenixMotorControlDevRef"=w431) -> ()  [unwired: 7 in, 2 out]
              }
            }
            n187 = case shown="True" w415 {
              tunnel: "H Med" -> [_ w433]
              tunnel: w411 -> [_ w432]
              frame False {
              }
              frame True {
                w440 = T10 0 items=["PercentOutput"=0, "Position"=1, "Velocity"=2, "Current"=3, "Follower"=5, "MotionProfile"=6, "MotionMagic"=7, "MotionProfileArc"=10, "Disabled"=15] ("Control Mode")
                n188 = call <vilib>:"CTRE_Phoenix_MotorControl_RefNumRegistryGet.vi"("refnum name"="Arm Actuator") -> ("PhoenixMotorControlDevRef"=w442:T3)  [unwired: 9 in, 1 out]
                n189 = Subtract(x=w433, y=70) -> (x-y=w436:i32)
                n190 = In Range and Coerce(upper limit=w433, x=w432, lower limit=w436) -> (In Range?=w435:bool)  [unwired: 1 out]
                n191 = Select(t=0.25 ("Output"), s=w435, f=1.0 ("Output")) -> (s? t:f=w434:dbl)
                n192 = call <vilib>:"CTRE_Phoenix_MotorControl_Set.vi"("Output"=w434, "Control Mode"=w440, "PhoenixMotorControlDevRef"=w442) -> ()  [unwired: 7 in, 2 out]
              }
            }
            n193 = Select(t=T1."Wait", s=w414, f=T1."H.Med") -> (s? t:f=w413:T1)
            n194 = call-poly <vilib>:"CTRE_Phoenix_MotorController_Get_Enhanced.vi"("PhoenixMotorControlDevRef"=w409) -> ("AnalogInRaw"=w412:i32)  [unwired: 10 in, 4 out]
          }
          frame "H.High" {
            # "Actual Position"
            # "Desired Position"
            # "Below"
            # "Neutral"
            # "Above"
            n195 = Add(x="H High", y=10) -> (x+y=w454:i32)
            n196 = Subtract(x="H High", y=10) -> (x-y=w455:i32)
            n197 = In Range and Coerce(upper limit=w454, x=w446, lower limit=w455) -> (In Range?=w451:bool)  [unwired: 1 out]
            n198 = Less?(x="H High", y=w446) -> (x < y?=w449:bool)
            n199 = Greater?(x="H High", y=w446) -> (0:w452:bool)
            n200 = case shown="True" w452 {
              tunnel: w446 -> [_ w469]
              tunnel: "H High" -> [_ w468]
              frame False {
              }
              frame True {
                w476 = T10 0 items=["PercentOutput"=0, "Position"=1, "Velocity"=2, "Current"=3, "Follower"=5, "MotionProfile"=6, "MotionMagic"=7, "MotionProfileArc"=10, "Disabled"=15] ("Control Mode")
                n201 = call <vilib>:"CTRE_Phoenix_MotorControl_RefNumRegistryGet.vi"("refnum name"="Arm Actuator") -> ("PhoenixMotorControlDevRef"=w478:T3)  [unwired: 9 in, 1 out]
                n202 = Subtract(x=w468, y=70) -> (x-y=w472:i32)
                n203 = In Range and Coerce(upper limit=w468, x=w469, lower limit=w472) -> (In Range?=w471:bool)  [unwired: 1 out]
                n204 = Select(t=0.25 ("Output"), s=w471, f=1.0 ("Output")) -> (s? t:f=w470:dbl)
                n205 = call <vilib>:"CTRE_Phoenix_MotorControl_Set.vi"("Output"=w470, "Control Mode"=w476, "PhoenixMotorControlDevRef"=w478) -> ()  [unwired: 7 in, 2 out]
              }
            }
            n206 = case shown="True" w449 {
              tunnel: w446 -> [_ w458]
              tunnel: "H High" -> [_ w457]
              frame False {
              }
              frame True {
                w465 = T10 0 items=["PercentOutput"=0, "Position"=1, "Velocity"=2, "Current"=3, "Follower"=5, "MotionProfile"=6, "MotionMagic"=7, "MotionProfileArc"=10, "Disabled"=15] ("Control Mode")
                n207 = call <vilib>:"CTRE_Phoenix_MotorControl_RefNumRegistryGet.vi"("refnum name"="Arm Actuator") -> ("PhoenixMotorControlDevRef"=w467:T3)  [unwired: 9 in, 1 out]
                n208 = Add(x=w457, y=70) -> (x+y=w462:i32)
                n209 = In Range and Coerce(upper limit=w462, x=w458, lower limit=w457) -> (In Range?=w460:bool)  [unwired: 1 out]
                n210 = Select(t=-0.25 ("Output"), s=w460, f=-1.0 ("Output")) -> (s? t:f=w459:dbl)
                n211 = call <vilib>:"CTRE_Phoenix_MotorControl_Set.vi"("Output"=w459, "Control Mode"=w465, "PhoenixMotorControlDevRef"=w467) -> ()  [unwired: 7 in, 2 out]
              }
            }
            n212 = Select(t=T1."Wait", s=w451, f=T1."H.High") -> (s? t:f=w450:T1)
            n213 = call-poly <vilib>:"CTRE_Phoenix_MotorController_Get_Enhanced.vi"("PhoenixMotorControlDevRef"=w447) -> ("AnalogInRaw"=w448:i32)  [unwired: 10 in, 4 out]
          }
          frame "C.Low" {
            # "Actual Position"
            # "Desired Position"
            # "Below"
            # "Neutral"
            # "Above"
            n214 = Add(x="C Low", y=10) -> (x+y=w490:i32)
            n215 = Subtract(x="C Low", y=10) -> (x-y=w491:i32)
            n216 = In Range and Coerce(upper limit=w490, x=w482, lower limit=w491) -> (In Range?=w487:bool)  [unwired: 1 out]
            n217 = Less?(x="C Low", y=w482) -> (x < y?=w486:bool)
            n218 = Greater?(x="C Low", y=w482) -> (0:w488:bool)
            n219 = case shown="True" w488 {
              tunnel: w482 -> [_ w505]
              tunnel: "C Low" -> [_ w504]
              frame False {
              }
              frame True {
                w512 = T10 0 items=["PercentOutput"=0, "Position"=1, "Velocity"=2, "Current"=3, "Follower"=5, "MotionProfile"=6, "MotionMagic"=7, "MotionProfileArc"=10, "Disabled"=15] ("Control Mode")
                n220 = call <vilib>:"CTRE_Phoenix_MotorControl_RefNumRegistryGet.vi"("refnum name"="Arm Actuator") -> ("PhoenixMotorControlDevRef"=w514:T3)  [unwired: 9 in, 1 out]
                n221 = Subtract(x=w504, y=70) -> (x-y=w508:i32)
                n222 = In Range and Coerce(upper limit=w504, x=w505, lower limit=w508) -> (In Range?=w507:bool)  [unwired: 1 out]
                n223 = Select(t=0.25 ("Output"), s=w507, f=1.0 ("Output")) -> (s? t:f=w506:dbl)
                n224 = call <vilib>:"CTRE_Phoenix_MotorControl_Set.vi"("Output"=w506, "Control Mode"=w512, "PhoenixMotorControlDevRef"=w514) -> ()  [unwired: 7 in, 2 out]
              }
            }
            n225 = case shown="True" w486 {
              tunnel: w482 -> [_ w494]
              tunnel: "C Low" -> [_ w493]
              frame False {
              }
              frame True {
                w501 = T10 0 items=["PercentOutput"=0, "Position"=1, "Velocity"=2, "Current"=3, "Follower"=5, "MotionProfile"=6, "MotionMagic"=7, "MotionProfileArc"=10, "Disabled"=15] ("Control Mode")
                n226 = call <vilib>:"CTRE_Phoenix_MotorControl_RefNumRegistryGet.vi"("refnum name"="Arm Actuator") -> ("PhoenixMotorControlDevRef"=w503:T3)  [unwired: 9 in, 1 out]
                n227 = Add(x=w493, y=70) -> (x+y=w498:i32)
                n228 = In Range and Coerce(upper limit=w498, x=w494, lower limit=w493) -> (In Range?=w496:bool)  [unwired: 1 out]
                n229 = Select(t=-0.25 ("Output"), s=w496, f=-1.0 ("Output")) -> (s? t:f=w495:dbl)
                n230 = call <vilib>:"CTRE_Phoenix_MotorControl_Set.vi"("Output"=w495, "Control Mode"=w501, "PhoenixMotorControlDevRef"=w503) -> ()  [unwired: 7 in, 2 out]
              }
            }
            n231 = Select(t=T1."Wait", s=w487, f=T1."C.Low") -> (s? t:f=w485:T1)
            n232 = call-poly <vilib>:"CTRE_Phoenix_MotorController_Get_Enhanced.vi"("PhoenixMotorControlDevRef"=w483) -> ("AnalogInRaw"=w484:i32)  [unwired: 10 in, 4 out]
          }
          frame "C.Med" {
            # "Actual Position"
            # "Desired Position"
            # "Below"
            # "Neutral"
            # "Above"
            n233 = Add(x="C Med", y=10) -> (x+y=w526:i32)
            n234 = Subtract(x="C Med", y=10) -> (x-y=w527:i32)
            n235 = In Range and Coerce(upper limit=w526, x=w518, lower limit=w527) -> (In Range?=w523:bool)  [unwired: 1 out]
            n236 = Less?(x="C Med", y=w518) -> (x < y?=w522:bool)
            n237 = Greater?(x="C Med", y=w518) -> (0:w524:bool)
            n238 = case shown="True" w524 {
              tunnel: w518 -> [_ w541]
              tunnel: "C Med" -> [_ w540]
              frame False {
              }
              frame True {
                w548 = T10 0 items=["PercentOutput"=0, "Position"=1, "Velocity"=2, "Current"=3, "Follower"=5, "MotionProfile"=6, "MotionMagic"=7, "MotionProfileArc"=10, "Disabled"=15] ("Control Mode")
                n239 = call <vilib>:"CTRE_Phoenix_MotorControl_RefNumRegistryGet.vi"("refnum name"="Arm Actuator") -> ("PhoenixMotorControlDevRef"=w550:T3)  [unwired: 9 in, 1 out]
                n240 = Subtract(x=w540, y=70) -> (x-y=w544:i32)
                n241 = In Range and Coerce(upper limit=w540, x=w541, lower limit=w544) -> (In Range?=w543:bool)  [unwired: 1 out]
                n242 = Select(t=0.25 ("Output"), s=w543, f=1.0 ("Output")) -> (s? t:f=w542:dbl)
                n243 = call <vilib>:"CTRE_Phoenix_MotorControl_Set.vi"("Output"=w542, "Control Mode"=w548, "PhoenixMotorControlDevRef"=w550) -> ()  [unwired: 7 in, 2 out]
              }
            }
            n244 = case shown="True" w522 {
              tunnel: w518 -> [_ w530]
              tunnel: "C Med" -> [_ w529]
              frame False {
              }
              frame True {
                w537 = T10 0 items=["PercentOutput"=0, "Position"=1, "Velocity"=2, "Current"=3, "Follower"=5, "MotionProfile"=6, "MotionMagic"=7, "MotionProfileArc"=10, "Disabled"=15] ("Control Mode")
                n245 = call <vilib>:"CTRE_Phoenix_MotorControl_RefNumRegistryGet.vi"("refnum name"="Arm Actuator") -> ("PhoenixMotorControlDevRef"=w539:T3)  [unwired: 9 in, 1 out]
                n246 = Add(x=w529, y=70) -> (x+y=w534:i32)
                n247 = In Range and Coerce(upper limit=w534, x=w530, lower limit=w529) -> (In Range?=w532:bool)  [unwired: 1 out]
                n248 = Select(t=-0.25 ("Output"), s=w532, f=-1.0 ("Output")) -> (s? t:f=w531:dbl)
                n249 = call <vilib>:"CTRE_Phoenix_MotorControl_Set.vi"("Output"=w531, "Control Mode"=w537, "PhoenixMotorControlDevRef"=w539) -> ()  [unwired: 7 in, 2 out]
              }
            }
            n250 = Select(t=T1."Wait", s=w523, f=T1."C.Med") -> (s? t:f=w521:T1)
            n251 = call-poly <vilib>:"CTRE_Phoenix_MotorController_Get_Enhanced.vi"("PhoenixMotorControlDevRef"=w519) -> ("AnalogInRaw"=w520:i32)  [unwired: 10 in, 4 out]
          }
          frame "C.High" {
            # "Actual Position"
            # "Desired Position"
            # "Below"
            # "Neutral"
            # "Above"
            n252 = Add(x="C High", y=10) -> (x+y=w562:i32)
            n253 = Subtract(x="C High", y=10) -> (x-y=w563:i32)
            n254 = In Range and Coerce(upper limit=w562, x=w554, lower limit=w563) -> (In Range?=w560:bool)  [unwired: 1 out]
            n255 = Less?(x="C High", y=w554) -> (x < y?=w557:bool)
            n256 = Greater?(x="C High", y=w554) -> (0:w558:bool)
            n257 = case shown="True" w557 {
              tunnel: w554 -> [_ w566]
              tunnel: "C High" -> [_ w565]
              frame False {
              }
              frame True {
                w573 = T10 0 items=["PercentOutput"=0, "Position"=1, "Velocity"=2, "Current"=3, "Follower"=5, "MotionProfile"=6, "MotionMagic"=7, "MotionProfileArc"=10, "Disabled"=15] ("Control Mode")
                n258 = call <vilib>:"CTRE_Phoenix_MotorControl_RefNumRegistryGet.vi"("refnum name"="Arm Actuator") -> ("PhoenixMotorControlDevRef"=w575:T3)  [unwired: 9 in, 1 out]
                n259 = Add(x=w565, y=70) -> (x+y=w570:i32)
                n260 = In Range and Coerce(upper limit=w570, x=w566, lower limit=w565) -> (In Range?=w568:bool)  [unwired: 1 out]
                n261 = Select(t=-0.25 ("Output"), s=w568, f=-1.0 ("Output")) -> (s? t:f=w567:dbl)
                n262 = call <vilib>:"CTRE_Phoenix_MotorControl_Set.vi"("Output"=w567, "Control Mode"=w573, "PhoenixMotorControlDevRef"=w575) -> ()  [unwired: 7 in, 2 out]
              }
            }
            n263 = case shown="True" w558 {
              tunnel: w554 -> [_ w577]
              tunnel: "C High" -> [_ w576]
              frame False {
              }
              frame True {
                w584 = T10 0 items=["PercentOutput"=0, "Position"=1, "Velocity"=2, "Current"=3, "Follower"=5, "MotionProfile"=6, "MotionMagic"=7, "MotionProfileArc"=10, "Disabled"=15] ("Control Mode")
                n264 = call <vilib>:"CTRE_Phoenix_MotorControl_RefNumRegistryGet.vi"("refnum name"="Arm Actuator") -> ("PhoenixMotorControlDevRef"=w586:T3)  [unwired: 9 in, 1 out]
                n265 = Subtract(x=w577, y=70) -> (x-y=w580:i32)
                n266 = In Range and Coerce(upper limit=w577, x=w576, lower limit=w580) -> (In Range?=w579:bool)  [unwired: 1 out]
                n267 = Select(t=0.25 ("Output"), s=w579, f=1.0 ("Output")) -> (s? t:f=w578:dbl)
                n268 = call <vilib>:"CTRE_Phoenix_MotorControl_Set.vi"("Output"=w578, "Control Mode"=w584, "PhoenixMotorControlDevRef"=w586) -> ()  [unwired: 7 in, 2 out]
              }
            }
            n269 = Select(t=T1."Wait", s=w560, f=T1."C.High") -> (s? t:f=w559:T1)
            n270 = call-poly <vilib>:"CTRE_Phoenix_MotorController_Get_Enhanced.vi"("PhoenixMotorControlDevRef"=w555) -> ("AnalogInRaw"=w556:i32)  [unwired: 10 in, 4 out]
          }
          frame "Home" {
            # "Bag Night Code = 0.4"
            # "Bag Night Code = -0.75"
            # "Bag Night Code = 0.4"
            # "Bag Night Code = 0.75"
            # "Actual Position"
            # "Desired Position"
            # "Below"
            # "Neutral"
            # "Above"
            n271 = Add(x="Home", y=18) -> (x+y=w598:i32)
            n272 = Subtract(x="Home", y=18) -> (x-y=w599:i32)
            n273 = In Range and Coerce(upper limit=w598, x=w590, lower limit=w599) -> (In Range?=w596:bool)  [unwired: 1 out]
            n274 = Less?(x="Home", y=w590) -> (x < y?=w594:bool)
            n275 = Greater?(x="Home", y=w590) -> (0:w595:bool)
            n276 = case shown="True" w595 {
              tunnel: w590 -> [_ w614]
              tunnel: "Home" -> [_ w613]
              frame False {
              }
              frame True {
                w620 = T10 0 items=["PercentOutput"=0, "Position"=1, "Velocity"=2, "Current"=3, "Follower"=5, "MotionProfile"=6, "MotionMagic"=7, "MotionProfileArc"=10, "Disabled"=15] ("Control Mode")
                n277 = call <vilib>:"CTRE_Phoenix_MotorControl_RefNumRegistryGet.vi"("refnum name"="Arm Actuator") -> ("PhoenixMotorControlDevRef"=w622:T3)  [unwired: 9 in, 1 out]
                n278 = Subtract(x=w613, y=50) -> (x-y=w616:i32)
                n279 = In Range and Coerce(upper limit=w613, x=w614, lower limit=w616) -> (In Range?=w615:bool)  [unwired: 1 out]
                n280 = Select(t=0.25 ("Output"), s=w615, f=0.5 ("Output")) -> (s? t:f=w612:dbl)
                n281 = call <vilib>:"CTRE_Phoenix_MotorControl_Set.vi"("Output"=w612, "Control Mode"=w620, "PhoenixMotorControlDevRef"=w622) -> ()  [unwired: 7 in, 2 out]
              }
            }
            n282 = case shown="True" w594 {
              tunnel: w590 -> [_ w602]
              tunnel: "Home" -> [_ w601]
              frame False {
              }
              frame True {
                w609 = T10 0 items=["PercentOutput"=0, "Position"=1, "Velocity"=2, "Current"=3, "Follower"=5, "MotionProfile"=6, "MotionMagic"=7, "MotionProfileArc"=10, "Disabled"=15] ("Control Mode")
                n283 = call <vilib>:"CTRE_Phoenix_MotorControl_RefNumRegistryGet.vi"("refnum name"="Arm Actuator") -> ("PhoenixMotorControlDevRef"=w611:T3)  [unwired: 9 in, 1 out]
                n284 = Add(x=w601, y=50) -> (x+y=w606:i32)
                n285 = In Range and Coerce(upper limit=w606, x=w602, lower limit=w601) -> (In Range?=w604:bool)  [unwired: 1 out]
                n286 = Select(t=-0.25 ("Output"), s=w604, f=-0.5 ("Output")) -> (s? t:f=w603:dbl)
                n287 = call <vilib>:"CTRE_Phoenix_MotorControl_Set.vi"("Output"=w603, "Control Mode"=w609, "PhoenixMotorControlDevRef"=w611) -> ()  [unwired: 7 in, 2 out]
              }
            }
            n288 = Select(t=T1."Wait", s=w596, f=T1."Home") -> (s? t:f=w593:T1)
            n289 = call-poly <vilib>:"CTRE_Phoenix_MotorController_Get_Enhanced.vi"("PhoenixMotorControlDevRef"=w591) -> ("AnalogInRaw"=w592:i32)  [unwired: 10 in, 4 out]
          }
          frame "Pull Out Grab" {
            # "Uses a sequence structure to move the claw up and backwards to pick up hatches"
            n290 = case shown="True" w628 {
              tunnel: w623 -> [_ w632]
              tunnel: w627 -> [w629 _]
              tunnel: [w629 w630] -> w626
              tunnel: w625 -> [_ w631]
              frame False {
              }
              frame True {
                n291 = flat-sequence {
                  tunnel: w632 -> [w634]
                  tunnel: w631 -> [w641]
                  tunnel: [T1."Wait"] -> w630
                  frame #0 {
                    # "Claw Up\nHigh enough to take the hatch."
                    n292 = for {
                      N: "Grab Time" -> [_]
                      tunnel: w634 -> [w638]
                      w637 = T10 0 items=["PercentOutput"=0, "Position"=1, "Velocity"=2, "Current"=3, "Follower"=5, "MotionProfile"=6, "MotionMagic"=7, "MotionProfileArc"=10, "Disabled"=15] ("Control Mode")
                      n293 = call <vilib>:"CTRE_Phoenix_MotorControl_Set.vi"("Output"=0.65, "Control Mode"=w637, "PhoenixMotorControlDevRef"=w638) -> ()  [unwired: 7 in, 2 out]
                      n294 = Wait (ms)(milliseconds to wait=u32 25) -> ()  [unwired: 1 out]
                    }
                  }
                  frame #1 {
                    n295 = for {
                      N: "Grab Wait Time" -> [_]
                      n296 = Wait (ms)(milliseconds to wait=u32 25) -> ()  [unwired: 1 out]
                    }
                  }
                  frame #2 {
                    # "Back Up\nFar enough to not interfere with the field."
                    n297 = for {
                      N: "Grab Drive Time" -> [_]
                      tunnel: w641 -> [w645]
                      # "Keep x, and rotation axies 0"
                      n298 = call-poly <vilib>:"WPI_RobotDriveHolonomicDrive.vi"("Rotation"=0.0, "Y"=0.5, "X"=0.0, "RobotDriveDevRef"=w645) -> ()  [unwired: 5 in, 3 out]
                      n299 = Wait (ms)(milliseconds to wait=u32 25) -> ()  [unwired: 1 out]
                    }
                  }
                  frame #3 {
                  }
                }
              }
            }
            n300 = call-poly <vilib>:"CTRE_Phoenix_MotorController_Get_Enhanced.vi"("PhoenixMotorControlDevRef"=w623) -> ("AnalogInRaw"=w624:i32)  [unwired: 10 in, 4 out]
          }
          frame "Pull Out Release" {
            # "Uses a sequence structure to move the claw down and backwards inorder to place the hatches"
            n301 = case shown="True" w653 {
              tunnel: w649 -> [_ w658]
              tunnel: w654 -> [w655 _]
              tunnel: [w655 w657] -> w652
              tunnel: w651 -> [_ w656]
              frame False {
              }
              frame True {
                n302 = flat-sequence {
                  tunnel: w658 -> [w661]
                  tunnel: w656 -> [w659]
                  tunnel: [T1."Wait"] -> w657
                  frame #0 {
                    # "Arm Down\nFar enough to let go of the hatch panel."
                    n303 = for {
                      N: "Release Time" -> [_]
                      tunnel: w661 -> [w669]
                      tunnel: w659 -> [w662]
                      w668 = T10 0 items=["PercentOutput"=0, "Position"=1, "Velocity"=2, "Current"=3, "Follower"=5, "MotionProfile"=6, "MotionMagic"=7, "MotionProfileArc"=10, "Disabled"=15] ("Control Mode")
                      # "Keep x, and rotation axies 0"
                      n304 = call-poly <vilib>:"WPI_RobotDriveHolonomicDrive.vi"("Rotation"=0.0, "Y"=0.5, "X"=0.0, "RobotDriveDevRef"=w662) -> ()  [unwired: 5 in, 3 out]
                      n305 = call <vilib>:"CTRE_Phoenix_MotorControl_Set.vi"("Output"=-0.55, "Control Mode"=w668, "PhoenixMotorControlDevRef"=w669) -> ()  [unwired: 7 in, 2 out]
                      n306 = Wait (ms)(milliseconds to wait=u32 25) -> ()  [unwired: 1 out]
                    }
                  }
                  frame #1 {
                  }
                }
              }
            }
            n307 = call-poly <vilib>:"CTRE_Phoenix_MotorController_Get_Enhanced.vi"("PhoenixMotorControlDevRef"=w649) -> ("AnalogInRaw"=w650:i32)  [unwired: 10 in, 4 out]
          }
          frame "Pre Climb" {
            # "Actual Position"
            # "Desired Position"
            # "Below"
            # "Neutral"
            # "Above"
            n308 = Add(x="Pre Climb", y=20) -> (x+y=w682:i32)
            n309 = Subtract(x="Pre Climb", y=20) -> (x-y=w683:i32)
            n310 = In Range and Coerce(upper limit=w682, x=w675, lower limit=w683) -> (In Range?=w678:bool)  [unwired: 1 out]
            n311 = Less?(x="Pre Climb", y=w675) -> (x < y?=w680:bool)
            n312 = Greater?(x="Pre Climb", y=w675) -> (0:w679:bool)
            n313 = case shown="True" w679 {
              tunnel: "Pre Climb" -> [_ w696]
              tunnel: w675 -> [_ w697]
              frame False {
              }
              frame True {
                w704 = T10 0 items=["PercentOutput"=0, "Position"=1, "Velocity"=2, "Current"=3, "Follower"=5, "MotionProfile"=6, "MotionMagic"=7, "MotionProfileArc"=10, "Disabled"=15] ("Control Mode")
                n314 = call <vilib>:"CTRE_Phoenix_MotorControl_RefNumRegistryGet.vi"("refnum name"="Arm Actuator") -> ("PhoenixMotorControlDevRef"=w706:T3)  [unwired: 9 in, 1 out]
                n315 = Subtract(x=w696, y=50) -> (x-y=w700:i32)
                n316 = In Range and Coerce(upper limit=w696, x=w697, lower limit=w700) -> (In Range?=w699:bool)  [unwired: 1 out]
                n317 = Select(t=0.25 ("Output"), s=w699, f=0.5 ("Output")) -> (s? t:f=w698:dbl)
                n318 = call <vilib>:"CTRE_Phoenix_MotorControl_Set.vi"("Output"=w698, "Control Mode"=w704, "PhoenixMotorControlDevRef"=w706) -> ()  [unwired: 7 in, 2 out]
              }
            }
            n319 = case shown="True" w680 {
              tunnel: "Pre Climb" -> [_ w685]
              tunnel: w675 -> [_ w686]
              frame False {
              }
              frame True {
                w693 = T10 0 items=["PercentOutput"=0, "Position"=1, "Velocity"=2, "Current"=3, "Follower"=5, "MotionProfile"=6, "MotionMagic"=7, "MotionProfileArc"=10, "Disabled"=15] ("Control Mode")
                n320 = call <vilib>:"CTRE_Phoenix_MotorControl_RefNumRegistryGet.vi"("refnum name"="Arm Actuator") -> ("PhoenixMotorControlDevRef"=w695:T3)  [unwired: 9 in, 1 out]
                n321 = Add(x=w685, y=50) -> (x+y=w689:i32)
                n322 = In Range and Coerce(upper limit=w689, x=w686, lower limit=w685) -> (In Range?=w687:bool)  [unwired: 1 out]
                n323 = Select(t=-0.25 ("Output"), s=w687, f=-0.5 ("Output")) -> (s? t:f=w692:dbl)
                n324 = call <vilib>:"CTRE_Phoenix_MotorControl_Set.vi"("Output"=w692, "Control Mode"=w693, "PhoenixMotorControlDevRef"=w695) -> ()  [unwired: 7 in, 2 out]
              }
            }
            n325 = Select(t=T1."Upward Travel", s=w678, f=T1."Pre Climb") -> (s? t:f=w674:T1)
            n326 = call-poly <vilib>:"CTRE_Phoenix_MotorController_Get_Enhanced.vi"("PhoenixMotorControlDevRef"=w676) -> ("AnalogInRaw"=w673:i32)  [unwired: 10 in, 4 out]
          }
          frame "Upward Travel" {
            # "Jack Foot"
            # "Jack"
            # "Arm"
            # "Uses the arm and jack to climb the habitat's side"
            n327 = for {
              N: 116 -> [_]
              tunnel: w715 -> [w729]
              tunnel: "Arm speed" -> [w728]
              tunnel: "Jack speed 1" -> [w727]
              tunnel: w712 -> [w726]
              tunnel: w711 -> [w722]
              tunnel: [w719] -> w708
              w723 = T10 0 items=["PercentOutput"=0, "Position"=1, "Velocity"=2, "Current"=3, "Follower"=5, "MotionProfile"=6, "MotionMagic"=7, "MotionProfileArc"=10, "Disabled"=15] ("Control Mode")
              w724 = T10 0 items=["PercentOutput"=0, "Position"=1, "Velocity"=2, "Current"=3, "Follower"=5, "MotionProfile"=6, "MotionMagic"=7, "MotionProfileArc"=10, "Disabled"=15] ("Control Mode")
              w725 = T10 0 items=["PercentOutput"=0, "Position"=1, "Velocity"=2, "Current"=3, "Follower"=5, "MotionProfile"=6, "MotionMagic"=7, "MotionProfileArc"=10, "Disabled"=15] ("Control Mode")
              n328 = call <vilib>:"CTRE_Phoenix_MotorControl_Set.vi"("Output"=w728, "Control Mode"=w724, "PhoenixMotorControlDevRef"=w729) -> ()  [unwired: 7 in, 2 out]
              n329 = call <vilib>:"CTRE_Phoenix_MotorControl_Set.vi"("Output"=w727, "Control Mode"=w725, "PhoenixMotorControlDevRef"=w726) -> ()  [unwired: 7 in, 2 out]
              n330 = call <vilib>:"CTRE_Phoenix_MotorControl_Set.vi"("Output"=0.0, "Control Mode"=w723, "PhoenixMotorControlDevRef"=w722) -> ("PhoenixMotorControlDevRef"=w719:T3)  [unwired: 7 in, 1 out]
              n331 = Wait (ms)(milliseconds to wait=u32 10) -> ()  [unwired: 1 out]
            }
            n332 = for {
              N: 1 -> [_]
              tunnel: [T1."Extra Jack Time"] -> w709
              tunnel: w708 -> [_]
              n333 = Wait (ms)(milliseconds to wait=u32 10) -> ()  [unwired: 1 out]
            }
          }
          frame "Extra Jack Time" {
            # "extra time given to jack the back end up to get more clearance on the platform"
            # "Jack Foot"
            # "Jack"
            # "Arm"
            n334 = for {
              N: 217 -> [_]
              tunnel: w737 -> [w751]
              tunnel: w736 -> [w750]
              tunnel: w735 -> [w749]
              tunnel: "Jack speed 2" -> [w745]
              tunnel: [w741] -> w732
              w746 = T10 0 items=["PercentOutput"=0, "Position"=1, "Velocity"=2, "Current"=3, "Follower"=5, "MotionProfile"=6, "MotionMagic"=7, "MotionProfileArc"=10, "Disabled"=15] ("Control Mode")
              w747 = T10 0 items=["PercentOutput"=0, "Position"=1, "Velocity"=2, "Current"=3, "Follower"=5, "MotionProfile"=6, "MotionMagic"=7, "MotionProfileArc"=10, "Disabled"=15] ("Control Mode")
              w748 = T10 0 items=["PercentOutput"=0, "Position"=1, "Velocity"=2, "Current"=3, "Follower"=5, "MotionProfile"=6, "MotionMagic"=7, "MotionProfileArc"=10, "Disabled"=15] ("Control Mode")
              n335 = call <vilib>:"CTRE_Phoenix_MotorControl_Set.vi"("Output"=0.0, "Control Mode"=w748, "PhoenixMotorControlDevRef"=w751) -> ()  [unwired: 7 in, 2 out]
              n336 = call <vilib>:"CTRE_Phoenix_MotorControl_Set.vi"("Output"=w745, "Control Mode"=w747, "PhoenixMotorControlDevRef"=w750) -> ()  [unwired: 7 in, 2 out]
              n337 = call <vilib>:"CTRE_Phoenix_MotorControl_Set.vi"("Output"=0.0, "Control Mode"=w746, "PhoenixMotorControlDevRef"=w749) -> ("PhoenixMotorControlDevRef"=w741:T3)  [unwired: 7 in, 1 out]
              n338 = Wait (ms)(milliseconds to wait=u32 10) -> ()  [unwired: 1 out]
            }
            n339 = for {
              N: 1 -> [_]
              tunnel: w732 -> [_]
              tunnel: [T1."Forward Travel"] -> w731
              n340 = Wait (ms)(milliseconds to wait=u32 10) -> ()  [unwired: 1 out]
            }
          }
          frame "Forward Travel" {
            # "Bring the robot forward onto the platform by running the jack foot"
            # "Jack Foot"
            # "Jack"
            # "Arm"
            n341 = for {
              N: 230 -> [_]
              tunnel: w759 -> [w773]
              tunnel: w758 -> [w772]
              tunnel: w757 -> [w771]
              tunnel: "Jack drive 1" -> [w767]
              tunnel: [w763] -> w752
              w768 = T10 0 items=["PercentOutput"=0, "Position"=1, "Velocity"=2, "Current"=3, "Follower"=5, "MotionProfile"=6, "MotionMagic"=7, "MotionProfileArc"=10, "Disabled"=15] ("Control Mode")
              w769 = T10 0 items=["PercentOutput"=0, "Position"=1, "Velocity"=2, "Current"=3, "Follower"=5, "MotionProfile"=6, "MotionMagic"=7, "MotionProfileArc"=10, "Disabled"=15] ("Control Mode")
              w770 = T10 0 items=["PercentOutput"=0, "Position"=1, "Velocity"=2, "Current"=3, "Follower"=5, "MotionProfile"=6, "MotionMagic"=7, "MotionProfileArc"=10, "Disabled"=15] ("Control Mode")
              n342 = Wait (ms)(milliseconds to wait=u32 10) -> ()  [unwired: 1 out]
              n343 = call <vilib>:"CTRE_Phoenix_MotorControl_Set.vi"("Output"=0.0, "Control Mode"=w769, "PhoenixMotorControlDevRef"=w773) -> ()  [unwired: 7 in, 2 out]
              n344 = call <vilib>:"CTRE_Phoenix_MotorControl_Set.vi"("Output"=0.0, "Control Mode"=w770, "PhoenixMotorControlDevRef"=w772) -> ()  [unwired: 7 in, 2 out]
              n345 = call <vilib>:"CTRE_Phoenix_MotorControl_Set.vi"("Output"=w767, "Control Mode"=w768, "PhoenixMotorControlDevRef"=w771) -> ("PhoenixMotorControlDevRef"=w763:T3)  [unwired: 7 in, 1 out]
            }
            n346 = for {
              N: 1 -> [_]
              tunnel: [T1."Jack Retrieval"] -> w754
              tunnel: w752 -> [_]
              n347 = Wait (ms)(milliseconds to wait=u32 10) -> ()  [unwired: 1 out]
            }
          }
          frame "Jack Retrieval" {
            # "bring the jack back up into the robot so we can be completely supported by the hab platform"
            # "Jack Foot"
            # "Jack"
            # "Arm"
            n348 = for {
              N: 325 -> [_]
              tunnel: w781 -> [w795]
              tunnel: w780 -> [w794]
              tunnel: w779 -> [w793]
              tunnel: "Jack speed 3" -> [w789]
              tunnel: [w785] -> w774
              w790 = T10 0 items=["PercentOutput"=0, "Position"=1, "Velocity"=2, "Current"=3, "Follower"=5, "MotionProfile"=6, "MotionMagic"=7, "MotionProfileArc"=10, "Disabled"=15] ("Control Mode")
              w791 = T10 0 items=["PercentOutput"=0, "Position"=1, "Velocity"=2, "Current"=3, "Follower"=5, "MotionProfile"=6, "MotionMagic"=7, "MotionProfileArc"=10, "Disabled"=15] ("Control Mode")
              w792 = T10 0 items=["PercentOutput"=0, "Position"=1, "Velocity"=2, "Current"=3, "Follower"=5, "MotionProfile"=6, "MotionMagic"=7, "MotionProfileArc"=10, "Disabled"=15] ("Control Mode")
              n349 = Wait (ms)(milliseconds to wait=u32 10) -> ()  [unwired: 1 out]
              n350 = call <vilib>:"CTRE_Phoenix_MotorControl_Set.vi"("Output"=0.0, "Control Mode"=w792, "PhoenixMotorControlDevRef"=w795) -> ()  [unwired: 7 in, 2 out]
              n351 = call <vilib>:"CTRE_Phoenix_MotorControl_Set.vi"("Output"=w789, "Control Mode"=w791, "PhoenixMotorControlDevRef"=w794) -> ()  [unwired: 7 in, 2 out]
              n352 = call <vilib>:"CTRE_Phoenix_MotorControl_Set.vi"("Output"=0.0, "Control Mode"=w790, "PhoenixMotorControlDevRef"=w793) -> ("PhoenixMotorControlDevRef"=w785:T3)  [unwired: 7 in, 1 out]
            }
            n353 = for {
              N: 1 -> [_]
              tunnel: [T1."Wait"] -> w776
              tunnel: w774 -> [_]
              n354 = Wait (ms)(milliseconds to wait=u32 10) -> ()  [unwired: 1 out]
            }
          }
          frame "Load Cargo" {
            # "Actual Position"
            # "Desired Position"
            # "Below"
            # "Neutral"
            # "Above"
            n355 = Add(x="Load Cargo", y=10) -> (x+y=w807:i32)
            n356 = Subtract(x="Load Cargo", y=10) -> (x-y=w808:i32)
            n357 = In Range and Coerce(upper limit=w807, x=w800, lower limit=w808) -> (In Range?=w803:bool)  [unwired: 1 out]
            n358 = Less?(x="Load Cargo", y=w800) -> (x < y?=w805:bool)
            n359 = Greater?(x="Load Cargo", y=w800) -> (0:w804:bool)
            n360 = case shown="True" w804 {
              tunnel: "Load Cargo" -> [_ w821]
              tunnel: w800 -> [_ w822]
              frame False {
              }
              frame True {
                w829 = T10 0 items=["PercentOutput"=0, "Position"=1, "Velocity"=2, "Current"=3, "Follower"=5, "MotionProfile"=6, "MotionMagic"=7, "MotionProfileArc"=10, "Disabled"=15] ("Control Mode")
                n361 = call <vilib>:"CTRE_Phoenix_MotorControl_RefNumRegistryGet.vi"("refnum name"="Arm Actuator") -> ("PhoenixMotorControlDevRef"=w831:T3)  [unwired: 9 in, 1 out]
                n362 = Subtract(x=w821, y=70) -> (x-y=w825:i32)
                n363 = In Range and Coerce(upper limit=w821, x=w822, lower limit=w825) -> (In Range?=w824:bool)  [unwired: 1 out]
                n364 = Select(t=0.25 ("Output"), s=w824, f=1.0 ("Output")) -> (s? t:f=w823:dbl)
                n365 = call <vilib>:"CTRE_Phoenix_MotorControl_Set.vi"("Output"=w823, "Control Mode"=w829, "PhoenixMotorControlDevRef"=w831) -> ()  [unwired: 7 in, 2 out]
              }
            }
            n366 = case shown="True" w805 {
              tunnel: "Load Cargo" -> [_ w810]
              tunnel: w800 -> [_ w811]
              frame False {
              }
              frame True {
                w818 = T10 0 items=["PercentOutput"=0, "Position"=1, "Velocity"=2, "Current"=3, "Follower"=5, "MotionProfile"=6, "MotionMagic"=7, "MotionProfileArc"=10, "Disabled"=15] ("Control Mode")
                n367 = call <vilib>:"CTRE_Phoenix_MotorControl_RefNumRegistryGet.vi"("refnum name"="Arm Actuator") -> ("PhoenixMotorControlDevRef"=w820:T3)  [unwired: 9 in, 1 out]
                n368 = Add(x=w810, y=70) -> (x+y=w814:i32)
                n369 = In Range and Coerce(upper limit=w814, x=w811, lower limit=w810) -> (In Range?=w812:bool)  [unwired: 1 out]
                n370 = Select(t=-0.25 ("Output"), s=w812, f=-1.0 ("Output")) -> (s? t:f=w817:dbl)
                n371 = call <vilib>:"CTRE_Phoenix_MotorControl_Set.vi"("Output"=w817, "Control Mode"=w818, "PhoenixMotorControlDevRef"=w820) -> ()  [unwired: 7 in, 2 out]
              }
            }
            n372 = Select(t=T1."Wait", s=w803, f=T1."Load Cargo") -> (s? t:f=w799:T1)
            n373 = call-poly <vilib>:"CTRE_Phoenix_MotorController_Get_Enhanced.vi"("PhoenixMotorControlDevRef"=w801) -> ("AnalogInRaw"=w798:i32)  [unwired: 10 in, 4 out]
          }
          frame "Pre Climb 2" {
            # "Change to \"Climb 2\" after testing"
            # "Actual Position"
            # "Desired Position"
            # "Below"
            # "Neutral"
            # "Above"
            n374 = Add(x="Pre Climb 2", y=20) -> (x+y=w843:i32)
            n375 = Subtract(x="Pre Climb 2", y=20) -> (x-y=w844:i32)
            n376 = In Range and Coerce(upper limit=w843, x=w835, lower limit=w844) -> (In Range?=w839:bool)  [unwired: 1 out]
            n377 = Less?(x="Pre Climb 2", y=w835) -> (x < y?=w841:bool)
            n378 = Greater?(x="Pre Climb 2", y=w835) -> (0:w840:bool)
            n379 = case shown="True" w840 {
              tunnel: "Pre Climb 2" -> [_ w857]
              tunnel: w835 -> [_ w858]
              frame False {
              }
              frame True {
                w865 = T10 0 items=["PercentOutput"=0, "Position"=1, "Velocity"=2, "Current"=3, "Follower"=5, "MotionProfile"=6, "MotionMagic"=7, "MotionProfileArc"=10, "Disabled"=15] ("Control Mode")
                n380 = call <vilib>:"CTRE_Phoenix_MotorControl_RefNumRegistryGet.vi"("refnum name"="Arm Actuator") -> ("PhoenixMotorControlDevRef"=w867:T3)  [unwired: 9 in, 1 out]
                n381 = Subtract(x=w857, y=50) -> (x-y=w861:i32)
                n382 = In Range and Coerce(upper limit=w857, x=w858, lower limit=w861) -> (In Range?=w860:bool)  [unwired: 1 out]
                n383 = Select(t=0.25 ("Output"), s=w860, f=0.5 ("Output")) -> (s? t:f=w859:dbl)
                n384 = call <vilib>:"CTRE_Phoenix_MotorControl_Set.vi"("Output"=w859, "Control Mode"=w865, "PhoenixMotorControlDevRef"=w867) -> ()  [unwired: 7 in, 2 out]
              }
            }
            n385 = case shown="True" w841 {
              tunnel: "Pre Climb 2" -> [_ w846]
              tunnel: w835 -> [_ w847]
              frame False {
              }
              frame True {
                w854 = T10 0 items=["PercentOutput"=0, "Position"=1, "Velocity"=2, "Current"=3, "Follower"=5, "MotionProfile"=6, "MotionMagic"=7, "MotionProfileArc"=10, "Disabled"=15] ("Control Mode")
                n386 = call <vilib>:"CTRE_Phoenix_MotorControl_RefNumRegistryGet.vi"("refnum name"="Arm Actuator") -> ("PhoenixMotorControlDevRef"=w856:T3)  [unwired: 9 in, 1 out]
                n387 = Add(x=w846, y=50) -> (x+y=w850:i32)
                n388 = In Range and Coerce(upper limit=w850, x=w847, lower limit=w846) -> (In Range?=w848:bool)  [unwired: 1 out]
                n389 = Select(t=-0.25 ("Output"), s=w848, f=-0.5 ("Output")) -> (s? t:f=w853:dbl)
                n390 = call <vilib>:"CTRE_Phoenix_MotorControl_Set.vi"("Output"=w853, "Control Mode"=w854, "PhoenixMotorControlDevRef"=w856) -> ()  [unwired: 7 in, 2 out]
              }
            }
            n391 = Select(t=T1."Upward Travel 2", s=w839, f=T1."Pre Climb 2") -> (s? t:f=w833:T1)
            n392 = call-poly <vilib>:"CTRE_Phoenix_MotorController_Get_Enhanced.vi"("PhoenixMotorControlDevRef"=w834) -> ("AnalogInRaw"=w832:i32)  [unwired: 10 in, 4 out]
          }
          frame "Upward Travel 2" {
            # "Uses the arm and jack to climb the habitat's side"
            # "593"
            n393 = for {
              N: 257 -> [_]
              tunnel: w875 -> [w883]
              tunnel: w874 -> [w890]
              tunnel: w873 -> [w889]
              tunnel: [w884] -> w876
              tunnel: "Arm speed-2" -> [w881]
              tunnel: "Jack speed 1-2" -> [w880]
              w886 = T10 0 items=["PercentOutput"=0, "Position"=1, "Velocity"=2, "Current"=3, "Follower"=5, "MotionProfile"=6, "MotionMagic"=7, "MotionProfileArc"=10, "Disabled"=15] ("Control Mode")
              w887 = T10 0 items=["PercentOutput"=0, "Position"=1, "Velocity"=2, "Current"=3, "Follower"=5, "MotionProfile"=6, "MotionMagic"=7, "MotionProfileArc"=10, "Disabled"=15] ("Control Mode")
              w888 = T10 0 items=["PercentOutput"=0, "Position"=1, "Velocity"=2, "Current"=3, "Follower"=5, "MotionProfile"=6, "MotionMagic"=7, "MotionProfileArc"=10, "Disabled"=15] ("Control Mode")
              n394 = call <vilib>:"CTRE_Phoenix_MotorControl_Set.vi"("Output"=w881, "Control Mode"=w887, "PhoenixMotorControlDevRef"=w883) -> ()  [unwired: 7 in, 2 out]
              n395 = call <vilib>:"CTRE_Phoenix_MotorControl_Set.vi"("Output"=w880, "Control Mode"=w888, "PhoenixMotorControlDevRef"=w890) -> ()  [unwired: 7 in, 2 out]
              n396 = call <vilib>:"CTRE_Phoenix_MotorControl_Set.vi"("Output"=0.0, "Control Mode"=w886, "PhoenixMotorControlDevRef"=w889) -> ("PhoenixMotorControlDevRef"=w884:T3)  [unwired: 7 in, 1 out]
              n397 = Wait (ms)(milliseconds to wait=u32 10) -> ()  [unwired: 1 out]
            }
            n398 = for {
              N: 1 -> [_]
              tunnel: [T1."Extra Jack Time 2"] -> w868
              tunnel: w876 -> [_]
              n399 = Wait (ms)(milliseconds to wait=u32 10) -> ()  [unwired: 1 out]
            }
          }
          frame "Extra Jack Time 2" {
            # "extra time given to jack the back end up to get more clearance on the platform"
            # "We may use this"
            n400 = for {
              N: 356 -> [_]
              tunnel: w897 -> [w912]
              tunnel: w896 -> [w911]
              tunnel: w895 -> [w910]
              tunnel: [w904] -> w898
              tunnel: "Jack speed 2-2" -> [w902]
              w907 = T10 0 items=["PercentOutput"=0, "Position"=1, "Velocity"=2, "Current"=3, "Follower"=5, "MotionProfile"=6, "MotionMagic"=7, "MotionProfileArc"=10, "Disabled"=15] ("Control Mode")
              w908 = T10 0 items=["PercentOutput"=0, "Position"=1, "Velocity"=2, "Current"=3, "Follower"=5, "MotionProfile"=6, "MotionMagic"=7, "MotionProfileArc"=10, "Disabled"=15] ("Control Mode")
              w909 = T10 0 items=["PercentOutput"=0, "Position"=1, "Velocity"=2, "Current"=3, "Follower"=5, "MotionProfile"=6, "MotionMagic"=7, "MotionProfileArc"=10, "Disabled"=15] ("Control Mode")
              n401 = call <vilib>:"CTRE_Phoenix_MotorControl_Set.vi"("Output"=0.0, "Control Mode"=w908, "PhoenixMotorControlDevRef"=w912) -> ()  [unwired: 7 in, 2 out]
              n402 = call <vilib>:"CTRE_Phoenix_MotorControl_Set.vi"("Output"=w902, "Control Mode"=w909, "PhoenixMotorControlDevRef"=w911) -> ()  [unwired: 7 in, 2 out]
              n403 = call <vilib>:"CTRE_Phoenix_MotorControl_Set.vi"("Output"=0.0, "Control Mode"=w907, "PhoenixMotorControlDevRef"=w910) -> ("PhoenixMotorControlDevRef"=w904:T3)  [unwired: 7 in, 1 out]
              n404 = Wait (ms)(milliseconds to wait=u32 10) -> ()  [unwired: 1 out]
            }
            n405 = for {
              N: 1 -> [_]
              tunnel: [T1."Forward Travel 2"] -> w891
              tunnel: w898 -> [_]
              n406 = Wait (ms)(milliseconds to wait=u32 10) -> ()  [unwired: 1 out]
            }
          }
          frame "Forward Travel 2" {
            # "Bring the robot forward onto the platform by running the jack foot"
            n407 = for {
              N: 230 -> [_]
              tunnel: w920 -> [w939]
              tunnel: w919 -> [w938]
              tunnel: w918 -> [w937]
              tunnel: [w930] -> w921
              tunnel: "Jack drive 1-2" -> [w929]
              tunnel: w913 -> [w928]
              w934 = T10 0 items=["PercentOutput"=0, "Position"=1, "Velocity"=2, "Current"=3, "Follower"=5, "MotionProfile"=6, "MotionMagic"=7, "MotionProfileArc"=10, "Disabled"=15] ("Control Mode")
              w935 = T10 0 items=["PercentOutput"=0, "Position"=1, "Velocity"=2, "Current"=3, "Follower"=5, "MotionProfile"=6, "MotionMagic"=7, "MotionProfileArc"=10, "Disabled"=15] ("Control Mode")
              w936 = T10 0 items=["PercentOutput"=0, "Position"=1, "Velocity"=2, "Current"=3, "Follower"=5, "MotionProfile"=6, "MotionMagic"=7, "MotionProfileArc"=10, "Disabled"=15] ("Control Mode")
              n408 = call <vilib>:"CTRE_Phoenix_MotorControl_Set.vi"("Output"=0.0, "Control Mode"=w935, "PhoenixMotorControlDevRef"=w939) -> ()  [unwired: 7 in, 2 out]
              n409 = call <vilib>:"CTRE_Phoenix_MotorControl_Set.vi"("Output"=0.0, "Control Mode"=w936, "PhoenixMotorControlDevRef"=w938) -> ()  [unwired: 7 in, 2 out]
              n410 = call <vilib>:"CTRE_Phoenix_MotorControl_Set.vi"("Output"=w929, "Control Mode"=w934, "PhoenixMotorControlDevRef"=w937) -> ("PhoenixMotorControlDevRef"=w930:T3)  [unwired: 7 in, 1 out]
              n411 = call-poly <vilib>:"WPI_RobotDriveHolonomicDrive.vi"("Rotation"=0.0, "Y"=-0.05, "X"=0.0, "RobotDriveDevRef"=w928) -> ()  [unwired: 5 in, 3 out]
              n412 = Wait (ms)(milliseconds to wait=u32 10) -> ()  [unwired: 1 out]
            }
            n413 = for {
              N: 1 -> [_]
              tunnel: [T1."Jack Retrieval 2"] -> w914
              tunnel: w921 -> [_]
              n414 = Wait (ms)(milliseconds to wait=u32 10) -> ()  [unwired: 1 out]
            }
          }
          frame "Jack Retrieval 2" {
            # "bring the jack back up into the robot so we can be completely supported by the hab platform"
            # "This only needs to go up\nfor very little time"
            n415 = for {
              N: 50 -> [_]
              tunnel: w946 -> [w961]
              tunnel: w945 -> [w960]
              tunnel: w944 -> [w959]
              tunnel: [w953] -> w947
              tunnel: "Jack speed 3-2" -> [w951]
              w956 = T10 0 items=["PercentOutput"=0, "Position"=1, "Velocity"=2, "Current"=3, "Follower"=5, "MotionProfile"=6, "MotionMagic"=7, "MotionProfileArc"=10, "Disabled"=15] ("Control Mode")
              w957 = T10 0 items=["PercentOutput"=0, "Position"=1, "Velocity"=2, "Current"=3, "Follower"=5, "MotionProfile"=6, "MotionMagic"=7, "MotionProfileArc"=10, "Disabled"=15] ("Control Mode")
              w958 = T10 0 items=["PercentOutput"=0, "Position"=1, "Velocity"=2, "Current"=3, "Follower"=5, "MotionProfile"=6, "MotionMagic"=7, "MotionProfileArc"=10, "Disabled"=15] ("Control Mode")
              n416 = call <vilib>:"CTRE_Phoenix_MotorControl_Set.vi"("Output"=0.0, "Control Mode"=w957, "PhoenixMotorControlDevRef"=w961) -> ()  [unwired: 7 in, 2 out]
              n417 = call <vilib>:"CTRE_Phoenix_MotorControl_Set.vi"("Output"=w951, "Control Mode"=w958, "PhoenixMotorControlDevRef"=w960) -> ()  [unwired: 7 in, 2 out]
              n418 = call <vilib>:"CTRE_Phoenix_MotorControl_Set.vi"("Output"=0.0, "Control Mode"=w956, "PhoenixMotorControlDevRef"=w959) -> ("PhoenixMotorControlDevRef"=w953:T3)  [unwired: 7 in, 1 out]
              n419 = Wait (ms)(milliseconds to wait=u32 10) -> ()  [unwired: 1 out]
            }
            n420 = for {
              N: 1 -> [_]
              tunnel: w947 -> [_]
              tunnel: [T1."Wait"] -> w940
              n421 = Wait (ms)(milliseconds to wait=u32 10) -> ()  [unwired: 1 out]
            }
          }
        }
      }
    }
  }
  n422 = disable-structure shown="Disabled" {
    frame Disabled {
      n423 = case shown="True" {
        selector: _ -> [_ _]
        tunnel: [w962 w990] -> _
        tunnel: _ -> [w962 _]
        frame False {
        }
        frame True {
          # "wait"
          # "Run the jack in the opposite direction\nto bring it into the robot and to allow \nforward movement all the way onto the platform"
          # "wait"
          # "Give power to jack foot to bring\nthe robot forward onto the platform"
          # "wait"
          # "Bring the back end of the robot\nfarther up, so it is safer to drive forward"
          # "Let the jack down and a little\npower for the arm to maintain level"
          # "98 Position for arm to go to"
          n424 = for {
            N: 50 -> [_]
            tunnel: _ -> [w1003]
            tunnel: _ -> [w1002]
            tunnel: _ -> [w1001]
            tunnel: [w994] -> w963
            tunnel: [w993] -> w964
            tunnel: [w992] -> w965
            w997 = T10 0 items=["PercentOutput"=0, "Position"=1, "Velocity"=2, "Current"=3, "Follower"=5, "MotionProfile"=6, "MotionMagic"=7, "MotionProfileArc"=10, "Disabled"=15] ("Control Mode")
            w999 = T10 0 items=["PercentOutput"=0, "Position"=1, "Velocity"=2, "Current"=3, "Follower"=5, "MotionProfile"=6, "MotionMagic"=7, "MotionProfileArc"=10, "Disabled"=15] ("Control Mode")
            w1000 = T10 0 items=["PercentOutput"=0, "Position"=1, "Velocity"=2, "Current"=3, "Follower"=5, "MotionProfile"=6, "MotionMagic"=7, "MotionProfileArc"=10, "Disabled"=15] ("Control Mode")
            n425 = Wait (ms)(milliseconds to wait=u32 10) -> ()  [unwired: 1 out]
            n426 = call <vilib>:"CTRE_Phoenix_MotorControl_Set.vi"("Output"=0.0, "Control Mode"=w997, "PhoenixMotorControlDevRef"=w1002) -> ("PhoenixMotorControlDevRef"=w992:T3)  [unwired: 7 in, 1 out]
            n427 = call <vilib>:"CTRE_Phoenix_MotorControl_Set.vi"("Output"=0.0, "Control Mode"=w999, "PhoenixMotorControlDevRef"=w1003) -> ("PhoenixMotorControlDevRef"=w993:T3)  [unwired: 7 in, 1 out]
            n428 = call <vilib>:"CTRE_Phoenix_MotorControl_Set.vi"("Output"=0.0, "Control Mode"=w1000, "PhoenixMotorControlDevRef"=w1001) -> ("PhoenixMotorControlDevRef"=w994:T3)  [unwired: 7 in, 1 out]
          }
          n429 = for {
            N: 116 -> [_]
            tunnel: w963 -> [w1075]
            tunnel: w964 -> [w1074]
            tunnel: [w1073] -> w989
            tunnel: [w1069] -> w987
            tunnel: w965 -> [w1068]
            tunnel: [w1066] -> w986
            w1070 = T10 0 items=["PercentOutput"=0, "Position"=1, "Velocity"=2, "Current"=3, "Follower"=5, "MotionProfile"=6, "MotionMagic"=7, "MotionProfileArc"=10, "Disabled"=15] ("Control Mode")
            w1071 = T10 0 items=["PercentOutput"=0, "Position"=1, "Velocity"=2, "Current"=3, "Follower"=5, "MotionProfile"=6, "MotionMagic"=7, "MotionProfileArc"=10, "Disabled"=15] ("Control Mode")
            w1072 = T10 0 items=["PercentOutput"=0, "Position"=1, "Velocity"=2, "Current"=3, "Follower"=5, "MotionProfile"=6, "MotionMagic"=7, "MotionProfileArc"=10, "Disabled"=15] ("Control Mode")
            n430 = Wait (ms)(milliseconds to wait=u32 10) -> ()  [unwired: 1 out]
            n431 = call <vilib>:"CTRE_Phoenix_MotorControl_Set.vi"("Control Mode"=w1071, "PhoenixMotorControlDevRef"=w1074) -> ("PhoenixMotorControlDevRef"=w1073:T3)  [unwired: 8 in, 1 out]
            n432 = call <vilib>:"CTRE_Phoenix_MotorControl_Set.vi"("Control Mode"=w1072, "PhoenixMotorControlDevRef"=w1075) -> ("PhoenixMotorControlDevRef"=w1069:T3)  [unwired: 8 in, 1 out]
            n433 = call <vilib>:"CTRE_Phoenix_MotorControl_Set.vi"("Output"=0.0, "Control Mode"=w1070, "PhoenixMotorControlDevRef"=w1068) -> ("PhoenixMotorControlDevRef"=w1066:T3)  [unwired: 7 in, 1 out]
          }
          n434 = for {
            N: 217 -> [_]
            tunnel: w989 -> [w1063]
            tunnel: [w1062] -> w988
            tunnel: w987 -> [w1058]
            tunnel: w986 -> [w1056]
            tunnel: [w1054] -> w985
            tunnel: [w1053] -> w984
            w1059 = T10 0 items=["PercentOutput"=0, "Position"=1, "Velocity"=2, "Current"=3, "Follower"=5, "MotionProfile"=6, "MotionMagic"=7, "MotionProfileArc"=10, "Disabled"=15] ("Control Mode")
            w1060 = T10 0 items=["PercentOutput"=0, "Position"=1, "Velocity"=2, "Current"=3, "Follower"=5, "MotionProfile"=6, "MotionMagic"=7, "MotionProfileArc"=10, "Disabled"=15] ("Control Mode")
            w1061 = T10 0 items=["PercentOutput"=0, "Position"=1, "Velocity"=2, "Current"=3, "Follower"=5, "MotionProfile"=6, "MotionMagic"=7, "MotionProfileArc"=10, "Disabled"=15] ("Control Mode")
            n435 = Wait (ms)(milliseconds to wait=u32 10) -> ()  [unwired: 1 out]
            n436 = call <vilib>:"CTRE_Phoenix_MotorControl_Set.vi"("Control Mode"=w1059, "PhoenixMotorControlDevRef"=w1063) -> ("PhoenixMotorControlDevRef"=w1062:T3)  [unwired: 8 in, 1 out]
            n437 = call <vilib>:"CTRE_Phoenix_MotorControl_Set.vi"("Output"=0.0, "Control Mode"=w1060, "PhoenixMotorControlDevRef"=w1056) -> ("PhoenixMotorControlDevRef"=w1054:T3)  [unwired: 7 in, 1 out]
            n438 = call <vilib>:"CTRE_Phoenix_MotorControl_Set.vi"("Output"=0.0, "Control Mode"=w1061, "PhoenixMotorControlDevRef"=w1058) -> ("PhoenixMotorControlDevRef"=w1053:T3)  [unwired: 7 in, 1 out]
          }
          n439 = for {
            N: 40 -> [_]
            tunnel: w988 -> [w1051]
            tunnel: w985 -> [w1050]
            tunnel: w984 -> [w1049]
            tunnel: [w1042] -> w983
            tunnel: [w1041] -> w982
            tunnel: [w1040] -> w981
            w1045 = T10 0 items=["PercentOutput"=0, "Position"=1, "Velocity"=2, "Current"=3, "Follower"=5, "MotionProfile"=6, "MotionMagic"=7, "MotionProfileArc"=10, "Disabled"=15] ("Control Mode")
            w1047 = T10 0 items=["PercentOutput"=0, "Position"=1, "Velocity"=2, "Current"=3, "Follower"=5, "MotionProfile"=6, "MotionMagic"=7, "MotionProfileArc"=10, "Disabled"=15] ("Control Mode")
            w1048 = T10 0 items=["PercentOutput"=0, "Position"=1, "Velocity"=2, "Current"=3, "Follower"=5, "MotionProfile"=6, "MotionMagic"=7, "MotionProfileArc"=10, "Disabled"=15] ("Control Mode")
            n440 = Wait (ms)(milliseconds to wait=u32 10) -> ()  [unwired: 1 out]
            n441 = call <vilib>:"CTRE_Phoenix_MotorControl_Set.vi"("Output"=0.0, "Control Mode"=w1045, "PhoenixMotorControlDevRef"=w1050) -> ("PhoenixMotorControlDevRef"=w1040:T3)  [unwired: 7 in, 1 out]
            n442 = call <vilib>:"CTRE_Phoenix_MotorControl_Set.vi"("Output"=0.0, "Control Mode"=w1047, "PhoenixMotorControlDevRef"=w1051) -> ("PhoenixMotorControlDevRef"=w1041:T3)  [unwired: 7 in, 1 out]
            n443 = call <vilib>:"CTRE_Phoenix_MotorControl_Set.vi"("Output"=0.0, "Control Mode"=w1048, "PhoenixMotorControlDevRef"=w1049) -> ("PhoenixMotorControlDevRef"=w1042:T3)  [unwired: 7 in, 1 out]
          }
          n444 = for {
            N: 230 -> [_]
            tunnel: w983 -> [w1035]
            tunnel: w982 -> [w1034]
            tunnel: w981 -> [w1033]
            tunnel: [w1030] -> w980
            tunnel: [w1029] -> w979
            tunnel: [w1028] -> w978
            w1036 = T10 0 items=["PercentOutput"=0, "Position"=1, "Velocity"=2, "Current"=3, "Follower"=5, "MotionProfile"=6, "MotionMagic"=7, "MotionProfileArc"=10, "Disabled"=15] ("Control Mode")
            w1037 = T10 0 items=["PercentOutput"=0, "Position"=1, "Velocity"=2, "Current"=3, "Follower"=5, "MotionProfile"=6, "MotionMagic"=7, "MotionProfileArc"=10, "Disabled"=15] ("Control Mode")
            w1038 = T10 0 items=["PercentOutput"=0, "Position"=1, "Velocity"=2, "Current"=3, "Follower"=5, "MotionProfile"=6, "MotionMagic"=7, "MotionProfileArc"=10, "Disabled"=15] ("Control Mode")
            n445 = Wait (ms)(milliseconds to wait=u32 10) -> ()  [unwired: 1 out]
            n446 = call <vilib>:"CTRE_Phoenix_MotorControl_Set.vi"("Control Mode"=w1036, "PhoenixMotorControlDevRef"=w1033) -> ("PhoenixMotorControlDevRef"=w1028:T3)  [unwired: 8 in, 1 out]
            n447 = call <vilib>:"CTRE_Phoenix_MotorControl_Set.vi"("Output"=0.0, "Control Mode"=w1037, "PhoenixMotorControlDevRef"=w1034) -> ("PhoenixMotorControlDevRef"=w1029:T3)  [unwired: 7 in, 1 out]
            n448 = call <vilib>:"CTRE_Phoenix_MotorControl_Set.vi"("Output"=0.0, "Control Mode"=w1038, "PhoenixMotorControlDevRef"=w1035) -> ("PhoenixMotorControlDevRef"=w1030:T3)  [unwired: 7 in, 1 out]
          }
          n449 = for {
            N: 80 -> [_]
            tunnel: w980 -> [w1023]
            tunnel: w979 -> [w1022]
            tunnel: w978 -> [w1021]
            tunnel: [w1017] -> w977
            tunnel: [w1016] -> w976
            tunnel: [w1015] -> w975
            w1024 = T10 0 items=["PercentOutput"=0, "Position"=1, "Velocity"=2, "Current"=3, "Follower"=5, "MotionProfile"=6, "MotionMagic"=7, "MotionProfileArc"=10, "Disabled"=15] ("Control Mode")
            w1025 = T10 0 items=["PercentOutput"=0, "Position"=1, "Velocity"=2, "Current"=3, "Follower"=5, "MotionProfile"=6, "MotionMagic"=7, "MotionProfileArc"=10, "Disabled"=15] ("Control Mode")
            w1026 = T10 0 items=["PercentOutput"=0, "Position"=1, "Velocity"=2, "Current"=3, "Follower"=5, "MotionProfile"=6, "MotionMagic"=7, "MotionProfileArc"=10, "Disabled"=15] ("Control Mode")
            n450 = Wait (ms)(milliseconds to wait=u32 10) -> ()  [unwired: 1 out]
            n451 = call <vilib>:"CTRE_Phoenix_MotorControl_Set.vi"("Output"=0.0, "Control Mode"=w1024, "PhoenixMotorControlDevRef"=w1021) -> ("PhoenixMotorControlDevRef"=w1015:T3)  [unwired: 7 in, 1 out]
            n452 = call <vilib>:"CTRE_Phoenix_MotorControl_Set.vi"("Output"=0.0, "Control Mode"=w1025, "PhoenixMotorControlDevRef"=w1022) -> ("PhoenixMotorControlDevRef"=w1017:T3)  [unwired: 7 in, 1 out]
            n453 = call <vilib>:"CTRE_Phoenix_MotorControl_Set.vi"("Output"=0.0, "Control Mode"=w1026, "PhoenixMotorControlDevRef"=w1023) -> ("PhoenixMotorControlDevRef"=w1016:T3)  [unwired: 7 in, 1 out]
          }
          n454 = for {
            N: 325 -> [_]
            tunnel: w977 -> [w1012]
            tunnel: w976 -> [w1007]
            tunnel: w975 -> [w1006]
            tunnel: [w1004] -> w968
            w1010 = T10 0 items=["PercentOutput"=0, "Position"=1, "Velocity"=2, "Current"=3, "Follower"=5, "MotionProfile"=6, "MotionMagic"=7, "MotionProfileArc"=10, "Disabled"=15] ("Control Mode")
            w1011 = T10 0 items=["PercentOutput"=0, "Position"=1, "Velocity"=2, "Current"=3, "Follower"=5, "MotionProfile"=6, "MotionMagic"=7, "MotionProfileArc"=10, "Disabled"=15] ("Control Mode")
            w1013 = T10 0 items=["PercentOutput"=0, "Position"=1, "Velocity"=2, "Current"=3, "Follower"=5, "MotionProfile"=6, "MotionMagic"=7, "MotionProfileArc"=10, "Disabled"=15] ("Control Mode")
            n455 = Wait (ms)(milliseconds to wait=u32 10) -> ()  [unwired: 1 out]
            n456 = call <vilib>:"CTRE_Phoenix_MotorControl_Set.vi"("Control Mode"=w1013, "PhoenixMotorControlDevRef"=w1012) -> ()  [unwired: 8 in, 2 out]
            n457 = call <vilib>:"CTRE_Phoenix_MotorControl_Set.vi"("Output"=0.0, "Control Mode"=w1010, "PhoenixMotorControlDevRef"=w1006) -> ("PhoenixMotorControlDevRef"=w1004:T3)  [unwired: 7 in, 1 out]
            n458 = call <vilib>:"CTRE_Phoenix_MotorControl_Set.vi"("Output"=0.0, "Control Mode"=w1011, "PhoenixMotorControlDevRef"=w1007) -> ()  [unwired: 7 in, 2 out]
          }
          n459 = for {
            N: 1 -> [_]
            tunnel: [_] -> w990
            tunnel: w968 -> [_]
            # "go to\nwait \ncase"
            n460 = Wait (ms)(milliseconds to wait=u32 10) -> ()  [unwired: 1 out]
          }
        }
      }
    }
    frame Enabled {
    }
  }
